vi "EC_Applied_Motion_SXSYSZ_20120115_3ch.vi"() -> ()   [LabVIEW 2015]
uses:
  <vilib>/Utility/file.llb/Read From Spreadsheet File (I64).vi
  <vilib>/Utility/file.llb/Read From Spreadsheet File (string).vi
  <vilib>/Instr/_visa.llb/VISA Configure Serial Port (Instr).vi
  <vilib>/Utility/file.llb/Write To Spreadsheet File (I64).vi
  <vilib>/Utility/file.llb/Write To Spreadsheet File (string).vi
panel:
  out "Z Velocity MV mm/sec":dbl format="%.3f"
  out "Z Position MV mm":dbl
  out "Y Velocity MV mm/sec":dbl format="%.3f"
  out "Y Position MV mm":dbl
  out "X Velocity MV mm/sec":dbl format="%.3f"
  out "X Position MV mm":dbl
  out "Presets":i32[][](array[numeric])
  in  "stop":bool
  in  "Tab Control 3":enum32{"Status", "Reset"}(tab)
  out "Y in Range":bool
  out "Y Scan":bool
  out "Y in Motion":bool
  out "Y Backlash corr":bool
  out "X  in Range":bool
  out "X Scan":bool
  out "X  in Motion":bool
  out "X Backlash corr":bool
  out "Z in Range":bool
  out "Z Scan":bool
  out "Z in Motion":bool
  out "Z Backlash corr":bool
  out "X Ready":bool
  out "Y Ready":bool
  out "Z Ready":bool
  in  "Reset Y Position mm":dbl
  out "Reset Y Motor Steps":i32
  in  "Reset X Position mm":dbl
  out "Reset X Motor Steps":i32
  in  "Reset Z Position mm":dbl
  out "Reset Z Motor Steps":i32
  in  "Reset":bool
  in  "Tab Control 2":enum32{"mm", "step"}(tab)
  in  "X Scan Length SP mm":dbl
  in  "X Scan Velocity SP mm/sec":dbl
  in  "X Scan set":bool
  in  "Y Scan Length SP mm":dbl
  in  "Y Scan Velocity SP mm/sec":dbl
  in  "Y Scan set":bool
  in  "Z Scan Length SP mm":dbl
  in  "Z Scan Velocity SP mm/sec":dbl
  in  "Z Scan set":bool
  in  "X Scan Velocity SP steps/sec":i32=1 min=1 max=102400 step=1
  in  "X Scan Length SP steps":i32 min=-500000 max=500000 step=100
  out "X Scan length MV mm":dbl
  out "X Scan velocity MV mm/sec":dbl format="%#_6f"
  in  "Y Scan Velocity SP steps/sec":i32=1 min=1 max=102400 step=1
  in  "Y Scan Length SP steps":i32 min=-1000000 max=0 step=100
  out "Y Scan length MV mm":dbl
  out "Y Scan velocity MV mm/sec":dbl format="%#_6f"
  in  "Z Scan Velocity SP steps/sec":i32=1 min=1 max=102400 step=1
  in  "Z Scan Length SP steps":i32 min=-204724 max=102195276 step=100
  out "Z Scan length MV mm":dbl
  out "Z Scan velocity MV mm/sec":dbl format="%#_6f"
  out "atan Y/Z":dbl
  in  "Tab Control":enum32{"mm", "preset", "step"}(tab)
  in  "X Position SP mm":dbl
  in  "X Velocity SP mm/sec":dbl
  in  "X Move Set":bool
  in  "Y Move Set":bool
  in  "Y Position SP mm":dbl
  in  "Y Velocity SP mm/sec":dbl
  in  "Z Position SP mm":dbl
  in  "Z Velocity SP mm/sec":dbl
  in  "Z Move Set":bool
  in  "Add Button":bool
  in  "String":string
  in  "Delete Button":bool
  in  "Preset positions":i32(ring) items=["ZERO", "Default", "CDOSE", "QMS", "test", "test2", "test3"]
  in  "Set Button":bool
  in  "X Velocity SP step/sec":i32 min=1 max=50000
  in  "Y Velocity SP step/sec":i32 min=1 max=50000
  in  "Z Velocity SP step/sec":i32 min=1 max=5000
  in  "Y Step SP":i32=-20000 min=-800000 max=800000 step=500
  in  "X Step SP":i32=-20000 min=-750000 max=750000 step=500
  in  "Z Step SP":i32=-20000 min=-3000 max=102400000 step=500
  out "X Step PV":i32 max=2000
  out "Y Step PV":i32 max=2000
  out "Z Step PV":i32 max=2000
  out "R Step PV":i32 max=2000
  out "X Scan Duration":dbl
  out "Y Scan Duration":dbl
  out "Z Scan Duration":dbl
  out "Z COM PORT":refnum<visa-resource-name>="COM5"
  out "Z Backlash steps/sec":i32
  out "Z Backlash":i32
  out "Z Holding Current %":i32
  out "Z Run Current %":i32
  out "Z offset mm":dbl
  out "Z mm/rev":dbl
  out "Z steps/rev":u32
  out "Z  velocity PV step/sec":i32
  out "Z MINPOS":i32=-94296
  out "Z MAXPOS":i32=-34296
  in  "Z Scan OK":bool
  in  "Z Go":bool
  out "Z Position mm PV":dbl
  out "X Position mm PV":dbl
  out "X velocity PV step/sec":i32
  in  "X Scan OK":bool
  in  "X Go":bool
  out "X Backlash steps/sec":i32
  out "X Backlash":i32
  out "X Holding Current %":i32
  out "X Run Current %":i32
  out "X offset mm":dbl
  out "X mm/rev":dbl
  out "X steps/rev":u32
  out "X MAXPOS":i32=-34296
  out "X MINPOS":i32=-94296
  out "X COM PORT":refnum<visa-resource-name>="COM5"
  out "Y Backlash steps/sec":i32
  out "Y Backlash":i32
  out "Y Holding Current %":i32
  out "Y Run Current %":i32
  in  "Scan Cancel":bool
  out "Y Position mm PV":dbl
  out "Y offset mm":dbl
  out "Y mm/rev":dbl
  out "Y steps/rev":u32
  out "Y velocity PV step/sec":i32
  in  "Y Scan OK":bool
  in  "Scan Go":bool
  in  "Stop":bool
  in  "Y Go":bool
  out "Y MINPOS":i32=-94296
  out "Y MAXPOS":i32=-34296
  out "Y COM PORT":refnum<visa-resource-name>="COM5"
  # "REF"
  # "Current position"
  # "Goto position"
  # "RX"
  # "RX"
  # "RY"
  # "RY"
  # "RZ"
  # "RZ"
  # "R,L = green"
  # "L"
  # "M"
  # "B"
  # "S"
  # "R"
  # "Preset position"
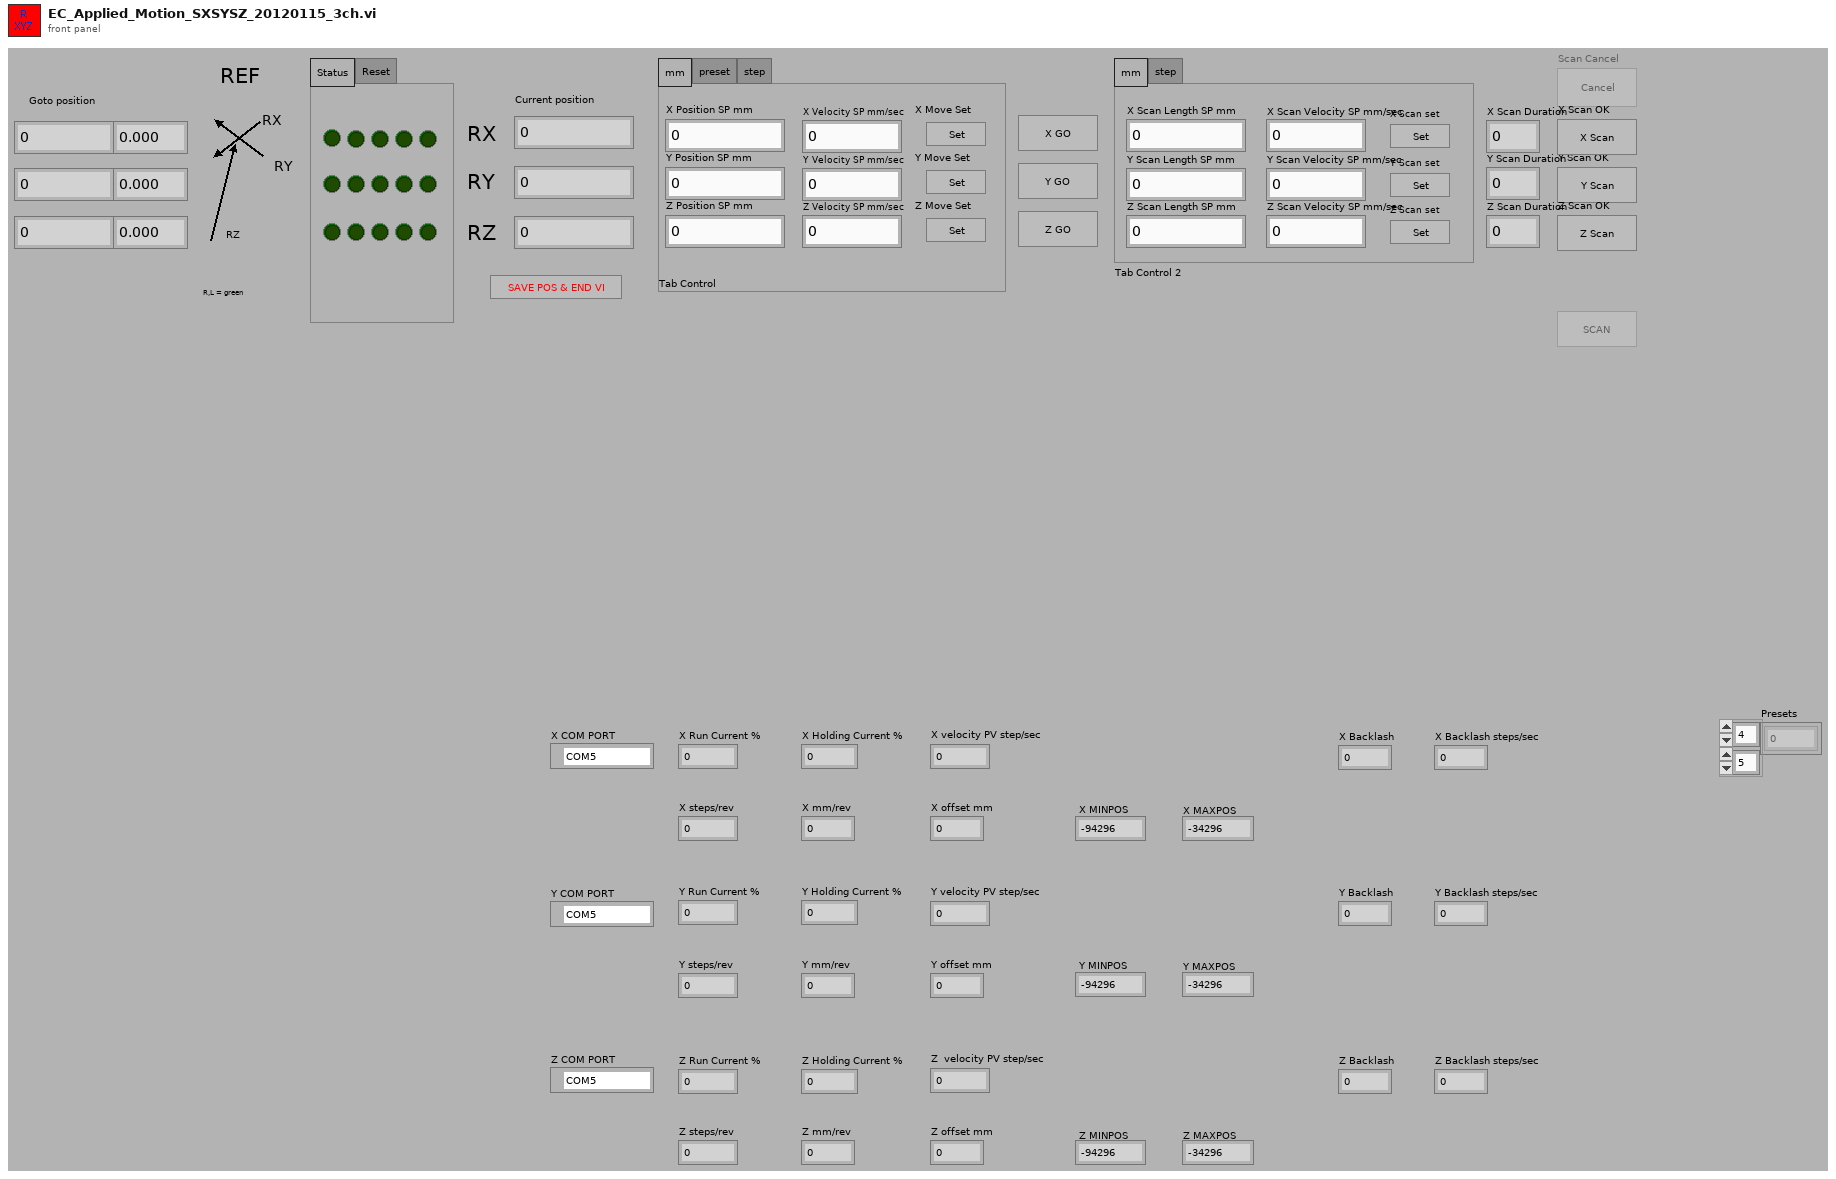
[diagram p1: front panel]
types:
  T1 = enum16{"Power-up Signature", "Accel Rate", "Accel Max", "Bit Rate", "Buffer Status", "Change Current", "Commence Jogging", "Change Jog Speed", "Continue", "Define Address", "Distance for FC,FM,FO,FY", "Decel Rate", "Distance or Position", "Define Limits", "Encoder Deadband", "Encoder Function", "Encoder Position", "Encoder Ratio", "Feed to Length with Speed Change", "Feed to Length", "Feed to Sensor with Mask Dist", "Feed to Length & Set Output", "Feed to Position", "Feed to Sensor", "Feed to Sensor w/safety", "Follow Handwheel", "Immediate Distance?", "Immediate Encoder?", "Immediate Low Output", "Immediate High Output", "Immediate Position?", "Input Status?", "Jog Accel/Decel", "Jog Disable", "Jog Enable", "Jog Speed", "Motor Disable", "Motor Enable", "Microstep Resolution", "Power up Current", "Power up Mode", "Pause", "Request Status", "Revision Level?", "Seek Home", "Stop Jogging", "Stop & Kill Buffer", "Set Output", "Set ABS Position", "Send String", "Stop", "Velocity for Speed Change", "Velocity Setting", "Wait for Input", "Wait Time"}
  T2 = enum8{"Enabled", "Disabled", "Disabled and Grayed Out"}
  T3 = cluster{"first row[0]":i64, "first row[1]":i64, "first row[2]":i64, "first row[3]":i64, "first row[4]":i64, "first row[5]":i64, "first row[6]":i64, "first row[7]":i64, "first row[8]":i64}
  T4 = cluster{"Value[0]":i32, "Value[1]":i32, "Value[2]":i32, "Value[3]":i32, "Value[4]":i32, "Value[5]":i32, "Value[6]":i32, "Value[7]":i32, "Value[8]":i32}
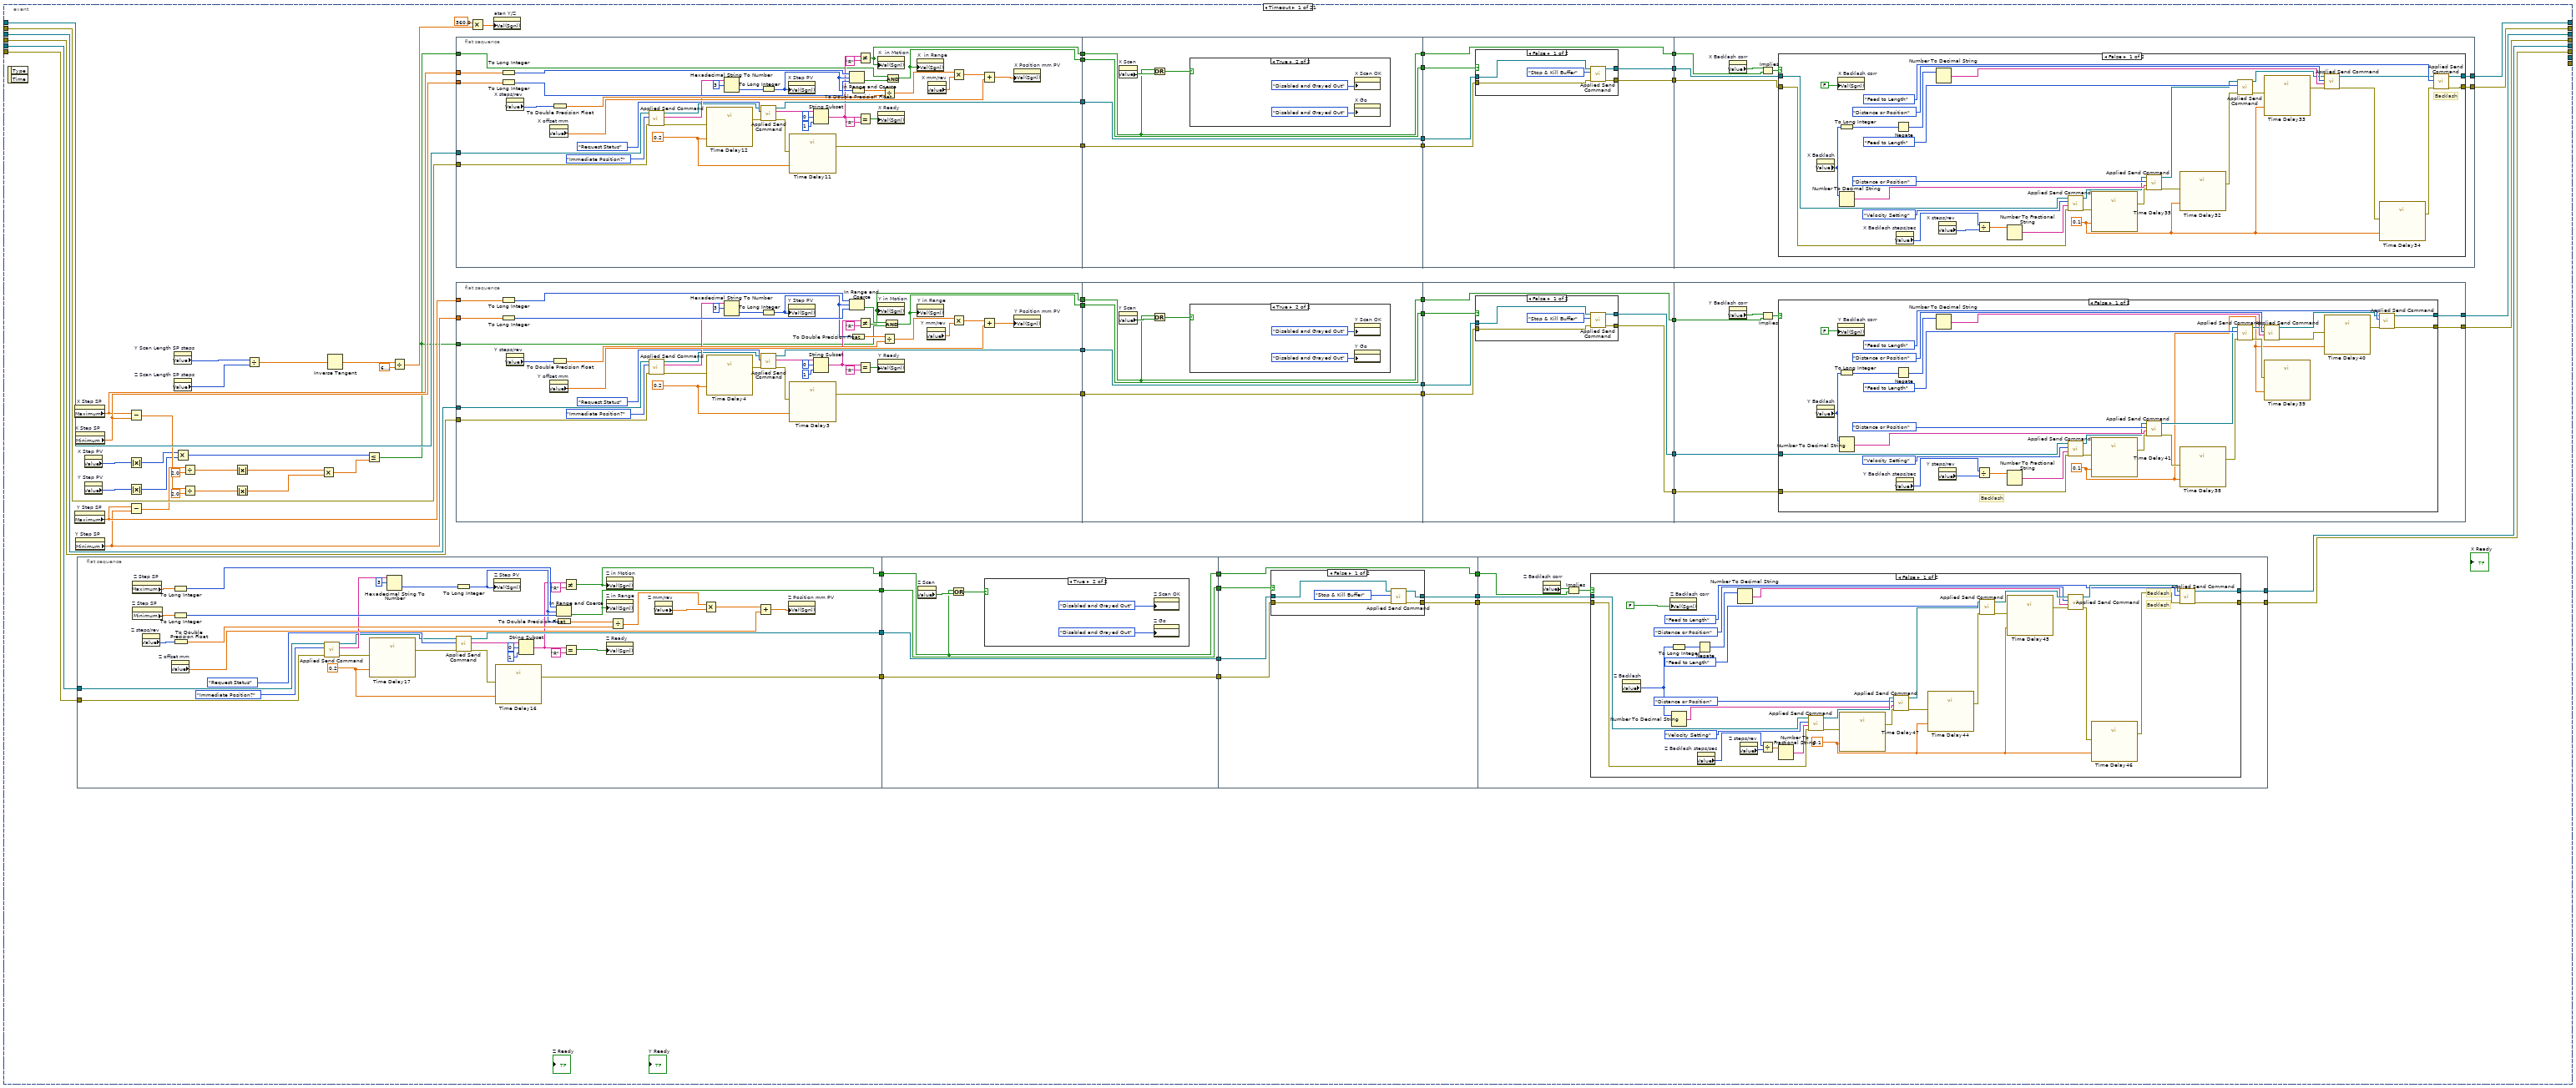
[diagram p5: hidden frame]
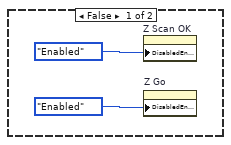
[diagram p6: hidden frame]
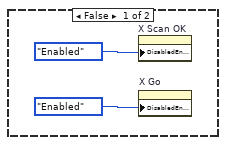
[diagram p9: hidden frame]
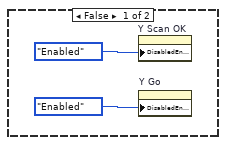
[diagram p12: hidden frame]
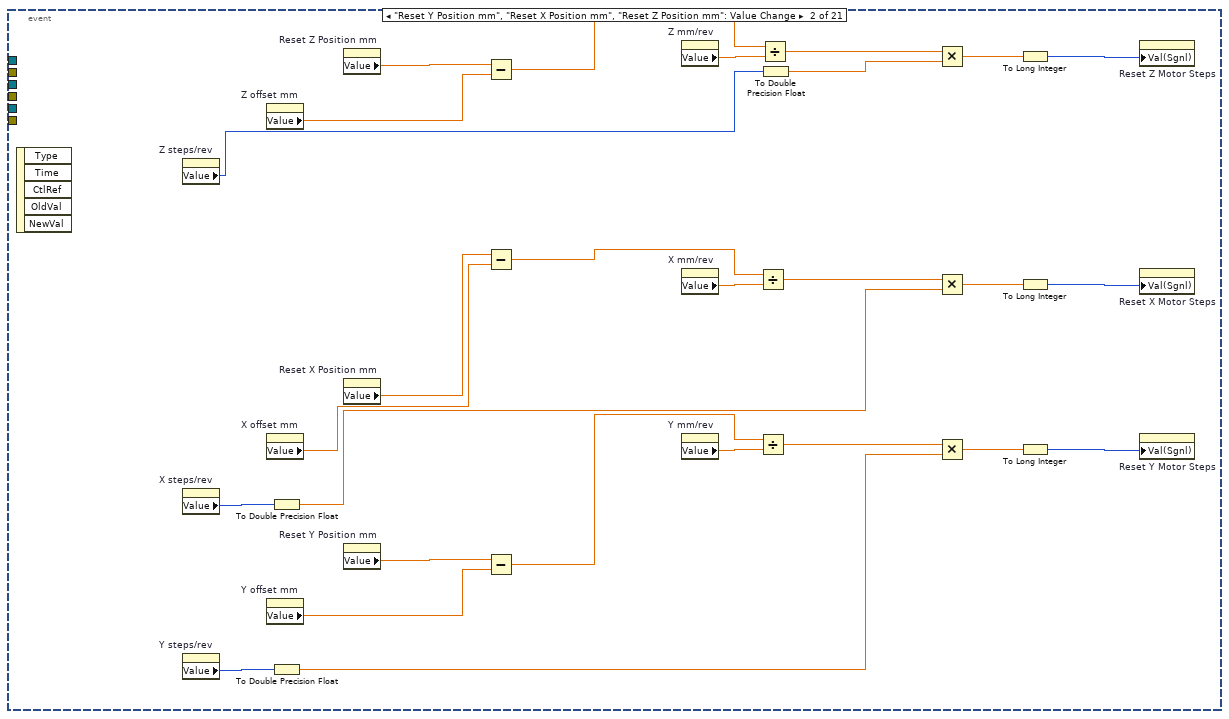
[diagram p15: hidden frame]
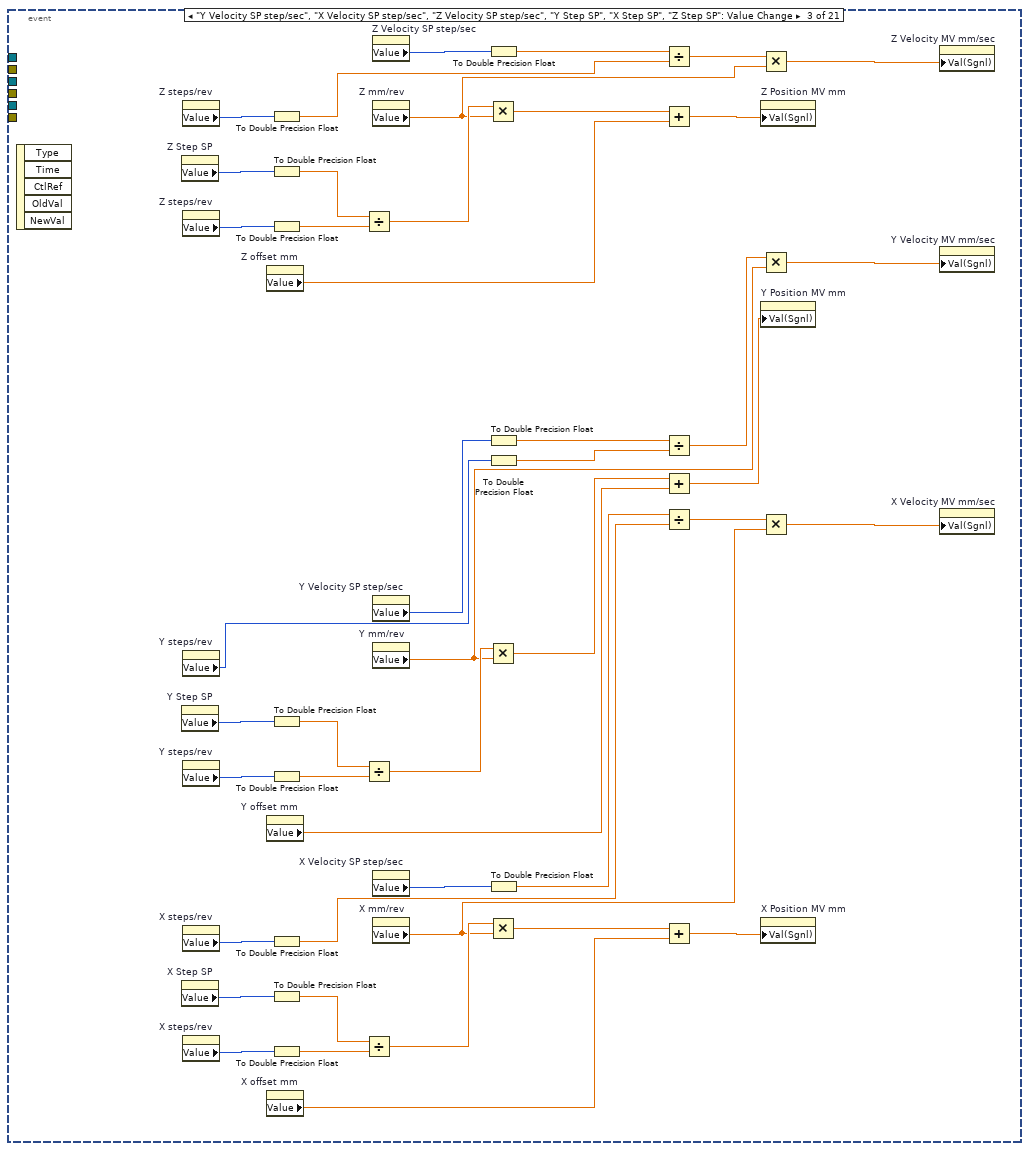
[diagram p16: hidden frame]
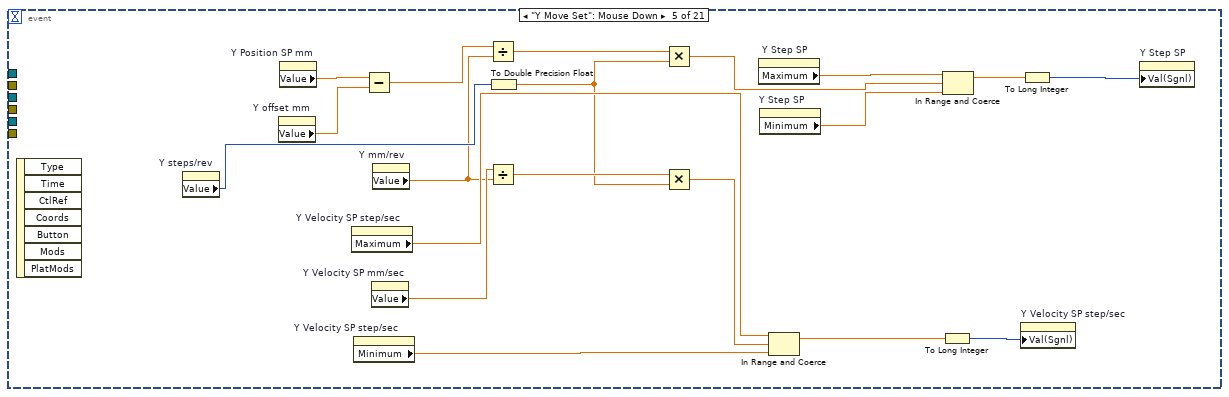
[diagram p17: hidden frame]
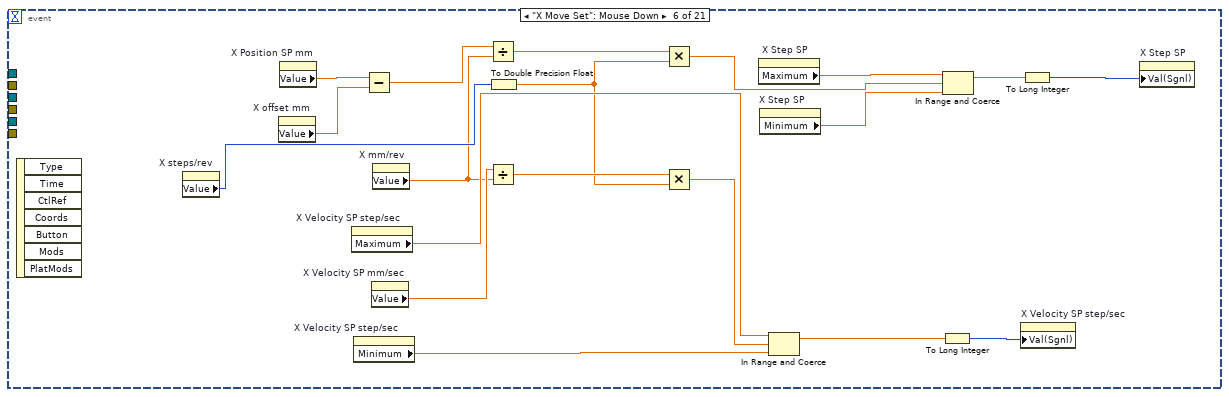
[diagram p18: hidden frame]
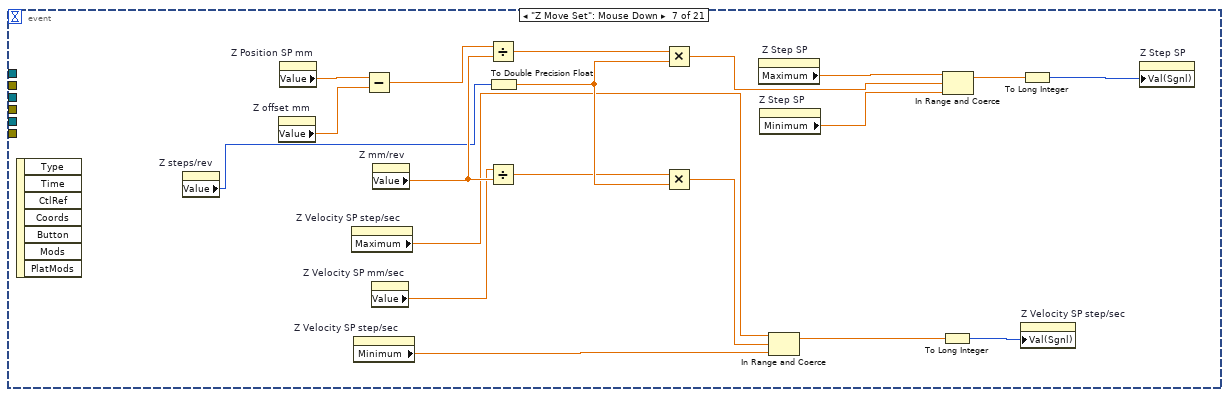
[diagram p19: hidden frame]
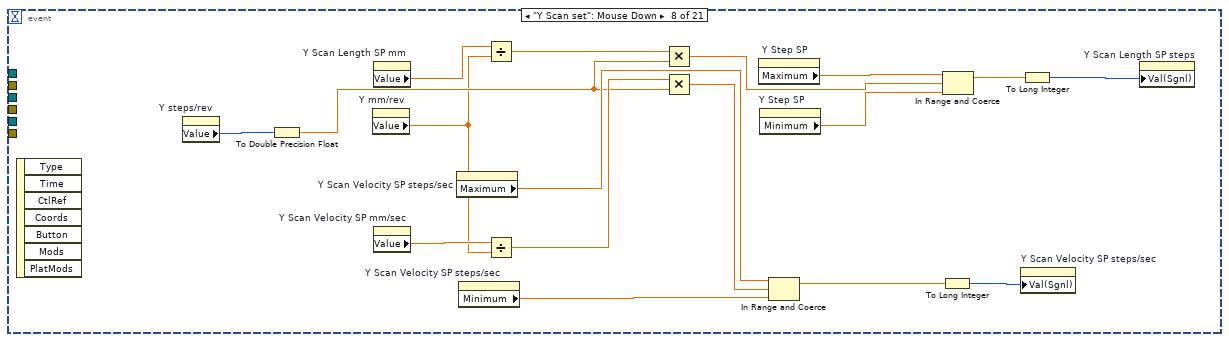
[diagram p20: hidden frame]
diagram:
  (unwired) FALSE
  w19 = 0 ("dimension size")
  n1 = flat-sequence {
    tunnel: [w78] -> w5
    tunnel: [w77] -> w4
    tunnel: w5 -> [w92]
    tunnel: w4 -> [w91]
    tunnel: [w90] -> w3
    tunnel: [w89] -> w2
    tunnel: [w100] -> w49
    tunnel: [w99] -> w48
    tunnel: w3 -> [w102]
    tunnel: w2 -> [w101]
    tunnel: w49 -> [w117]
    tunnel: w48 -> [w116]
    tunnel: [w118] -> w47
    tunnel: [w119] -> w46
    tunnel: [w120] -> w1
    tunnel: [w131] -> w44
    tunnel: [w132] -> w45
    tunnel: w47 -> [w132]
    tunnel: w46 -> [w131]
    tunnel: w1 -> [w129]
    frame #0 {
      "Z Run Current %" <- 100 ("Z Run Current %")
      "Z Holding Current %" <- 50 ("Z Holding Current %")
    }
    frame #1 {
      "Z Backlash steps/sec" <- 1000 ("Z Backlash steps/sec")
      "Z Backlash" <- -2500 ("Z Backlash")
    }
    frame #2 {
      w68 = 2.54 ("Z mm/rev")
      w67 = u32 20000 ("step/rev")
      w69 = 5000 ("Value (Signaling)")
      n2 = property on="Z Velocity SP step/sec" class="DigNum (strict)"("Minimum"=1.0 ("Data Entry Limits:Minimum")) -> ()  [unwired: 2 in, 2 out]
      n3 = property on="Z Scan Velocity SP mm/sec" class="DigNum (strict)"("Val(Sgnl)"=0.1 ("Value (Signaling)")) -> ()  [unwired: 2 in, 2 out]
      n4 = property on="Z Velocity SP step/sec" class="DigNum (strict)"("Val(Sgnl)"=w69) -> ()  [unwired: 2 in, 2 out]
      n5 = To Double Precision Float(number=w69) -> (double precision float=w73:dbl)
      n6 = property on="Z Velocity SP step/sec" class="DigNum (strict)"("Maximum"=w73) -> ()  [unwired: 2 in, 2 out]
      n7 = To Double Precision Float(number=w67) -> (double precision float=w72:dbl)
      n8 = Divide(x=w73, y=w72) -> (x/y=w70:dbl)
      n9 = Multiply(x=w70, y=w68) -> (x*y=w71:dbl)
      n10 = property on="Z Velocity SP mm/sec" class="DigNum (strict)"("Val(Sgnl)"=w71) -> ()  [unwired: 2 in, 2 out]
      "Z mm/rev" <- w68
      "Z steps/rev" <- w67
    }
    frame #3 {
      w75 = -3000 ("lower limit")
      w74 = 102400000 ("upper limit")
      n11 = property on="Z Step SP" class="DigNum (strict)"("Minimum"=w75) -> ()  [unwired: 2 in, 2 out]
      n12 = property on="Z Step SP" class="DigNum (strict)"("Maximum"=w74) -> ()  [unwired: 2 in, 2 out]
      "Z offset mm" <- 0.0 ("Z offset mm")
      "Z MINPOS" <- w75
      "Z MAXPOS" <- w74
    }
    frame #4 {
      w85 = refnum<visa-resource-name> "COM15" ("COM PORT")
      w83 = u16 0 items=["None", "XON/XOFF", "RTS/CTS", "XON/XOFF & RTS/CTS", "DTR/DSR", "XON/XOFF & DTR/DSR"] ("flow control (0:none)")
      w82 = u16 10 items=["1.0"=10, "1.5"=15, "2.0"=20] ("stop bits (10: 1 bit)")
      # "Stop bits"
      n13 = call-poly "VISA Configure Serial Port"("VISA resource name"=w85, "timeout (10sec)"=u32 10000, "baud rate (9600)"=u32 9600, "data bits (8)"=u16 8, "parity (0:none)"=enum16{"None", "Odd", "Even", "Mark", "Space"}."None", "stop bits (10: 1 bit)"=w82, "flow control (0:none)"=w83) -> ("VISA resource name out"=w78:refnum<visa-resource-name>, "error out"=w77:errorcluster)  [unwired: 7 in]
      "Z COM PORT" <- w85
    }
    frame #5 {
      # "Run Current %"
      n14 = property on="Z Run Current %" class="DigNum (strict)"() -> ("Value"=w93:i32)  [unwired: 2 in, 2 out]
      n15 = Divide(x=w93, y=100) -> (x/y=w94:dbl)
      n16 = Multiply(x=w94, y=3.5) -> (x*y=w88:dbl)
      n17 = Number To Fractional String(number=w88) -> (F-format string=w95:string)  [unwired: 3 in]
      n18 = call "Applied Send Command.vi"("error in (no error)"=w91, "Extra"=w95, "Command"=T1."Change Current", "VISA resource name"=w92) -> ("error out"=w89:errorcluster, "VISA resource name out"=w90:refnum<visa-resource-name>)  [unwired: 3 in, 1 out]
    }
    frame #6 {
      # "VELOCITY"
      n19 = property on="Z steps/rev" class="DigNum (strict)"() -> ("Value"=w98:u32)  [unwired: 2 in, 2 out]
      n20 = property on="Z Velocity SP step/sec" class="DigNum (strict)"() -> ("Value"=w97:i32)  [unwired: 2 in, 2 out]
      n21 = Divide(x=w97, y=w98) -> (x/y=w105:dbl)
      n22 = Number To Fractional String(number=w105) -> (F-format string=w107:string)  [unwired: 3 in]
      n23 = call "Applied Send Command.vi"("error in (no error)"=w101, "Extra"=w107, "Command"=T1."Velocity Setting", "VISA resource name"=w102) -> ("error out"=w108:errorcluster, "VISA resource name out"=w115:refnum<visa-resource-name>)  [unwired: 3 in, 1 out]
      n24 = call "Time Delay2"("error in (no error)"=w108, "Delay Time (s)"=0.1) -> ("error out"=w113:errorcluster)  [unwired: 9 in]
      n25 = call "Applied Send Command.vi"("error in (no error)"=w113, "Extra"="", "Command"=T1."Velocity Setting", "VISA resource name"=w115) -> ("error out"=w99:errorcluster, "read buffer"=w111:string, "VISA resource name out"=w100:refnum<visa-resource-name>)  [unwired: 3 in]
      n26 = Fract/Exp String To Number(string=w111, offset=3) -> (number=w106:dbl)  [unwired: 2 in, 1 out]
      n27 = Multiply(x=w106, y=w98) -> (x*y=w103:dbl)
      n28 = property on="Z  velocity PV step/sec" class="DigNum (strict)"("Val(Sgnl)"=w103) -> ()  [unwired: 2 in, 2 out]
    }
    frame #7 {
      # "GET CURRENT POSITION"
      n29 = call "Applied Send Command.vi"("error in (no error)"=w116, "Extra"="", "Command"=T1."Immediate Position?", "VISA resource name"=w117) -> ("error out"=w122:errorcluster, "read buffer"=w124:string, "VISA resource name out"=w118:refnum<visa-resource-name>)  [unwired: 3 in]
      n30 = call "Time Delay8"("error in (no error)"=w122, "Delay Time (s)"=0.1) -> ("error out"=w119:errorcluster)  [unwired: 9 in]
      n31 = Hexadecimal String To Number(string=w124, offset=3) -> (number=w120:u32)  [unwired: 1 in, 1 out]
    }
    frame #8 {
      n32 = property on="Z Step SP" class="DigNum (strict)"() -> ("Maximum"=w128:dbl)  [unwired: 2 in, 2 out]
      n33 = property on="Z Step SP" class="DigNum (strict)"() -> ("Minimum"=w127:dbl)  [unwired: 2 in, 2 out]
      n34 = property on="Z Step SP" class="DigNum (strict)"("Val(Sgnl)"=w129) -> ()  [unwired: 2 in, 2 out]
      n35 = In Range and Coerce(upper limit=w128, x=w129, lower limit=w127) -> (In Range?=w130:bool)  [unwired: 1 out]
      n36 = property on="Z in Range" class="Bool (strict)"("Val(Sgnl)"=w130) -> ()  [unwired: 2 in, 2 out]
    }
  }
  n37 = flat-sequence {
    frame #0 {
      n38 = property on="X Scan" class="Bool (strict)"("Val(Sgnl)"=FALSE ("Value (Signaling)")) -> ()  [unwired: 2 in, 2 out]
      n39 = property on="Y Scan" class="Bool (strict)"("Val(Sgnl)"=FALSE ("Value (Signaling)")) -> ()  [unwired: 2 in, 2 out]
      n40 = property on="Z Scan" class="Bool (strict)"("Val(Sgnl)"=FALSE ("Value (Signaling)")) -> ()  [unwired: 2 in, 2 out]
      n41 = property on="Scan Go" class="Bool"("DisabledEnum"=T2."Disabled and Grayed Out" ("Disabled")) -> ()  [unwired: 2 in, 2 out]
      n42 = property on="Scan Cancel" class="Bool"("DisabledEnum"=T2."Disabled and Grayed Out" ("Disabled")) -> ()  [unwired: 2 in, 2 out]
    }
    frame #1 {
      n43 = property on="Y Backlash corr" class="Bool (strict)"("Val(Sgnl)"=FALSE ("Value (Signaling)")) -> ()  [unwired: 2 in, 2 out]
      n44 = property on="X Backlash corr" class="Bool (strict)"("Val(Sgnl)"=FALSE ("Value (Signaling)")) -> ()  [unwired: 2 in, 2 out]
      n45 = property on="Z Backlash corr" class="Bool (strict)"("Val(Sgnl)"=FALSE ("Value (Signaling)")) -> ()  [unwired: 2 in, 2 out]
    }
  }
  n46 = flat-sequence {
    tunnel: [w158] -> w13
    tunnel: [w157] -> w12
    tunnel: w13 -> [w172]
    tunnel: w12 -> [w171]
    tunnel: [w170] -> w11
    tunnel: [w169] -> w10
    tunnel: w11 -> [w180]
    tunnel: w10 -> [w179]
    tunnel: [w178] -> w9
    tunnel: [w177] -> w8
    tunnel: [w197] -> w53
    tunnel: w9 -> [w200]
    tunnel: w8 -> [w199]
    tunnel: [w198] -> w7
    tunnel: [w196] -> w6
    tunnel: [w209] -> w59
    tunnel: [w212] -> w60
    tunnel: w53 -> [w209]
    tunnel: w7 -> [w212]
    tunnel: w6 -> [w210]
    frame #0 {
      "Y Run Current %" <- 100 ("Run Current %")
      "Y Holding Current %" <- 50 ("Holding Current %")
    }
    frame #1 {
      "Y Backlash" <- 5000 ("Backlash2")
      "Y Backlash steps/sec" <- 10000 ("Value (Signaling)")
    }
    frame #2 {
      w148 = 0.21167 ("MM/rev")
      w151 = u32 20000 ("step/rev")
      w146 = 50000 ("Value (Signaling)")
      n47 = property on="Y Velocity SP step/sec" class="DigNum (strict)"("Minimum"=1.0 ("Data Entry Limits:Minimum")) -> ()  [unwired: 2 in, 2 out]
      n48 = property on="Y Scan Velocity SP mm/sec" class="DigNum (strict)"("Val(Sgnl)"=0.1 ("Value (Signaling)")) -> ()  [unwired: 2 in, 2 out]
      n49 = property on="Y Velocity SP step/sec" class="DigNum (strict)"("Val(Sgnl)"=w146) -> ()  [unwired: 2 in, 2 out]
      n50 = To Double Precision Float(number=w146) -> (double precision float=w152:dbl)
      n51 = property on="Y Velocity SP step/sec" class="DigNum (strict)"("Maximum"=w152) -> ()  [unwired: 2 in, 2 out]
      n52 = To Double Precision Float(number=w151) -> (double precision float=w150:dbl)
      n53 = Divide(x=w152, y=w150) -> (x/y=w147:dbl)
      n54 = Multiply(x=w147, y=w148) -> (x*y=w149:dbl)
      n55 = property on="Y Velocity SP mm/sec" class="DigNum (strict)"("Val(Sgnl)"=w149) -> ()  [unwired: 2 in, 2 out]
      "Y steps/rev" <- w151
      "Y mm/rev" <- w148
    }
    frame #3 {
      w155 = -800000 ("lower limit")
      w156 = 800000 ("upper limit")
      n56 = property on="Y Step SP" class="DigNum (strict)"("Minimum"=w155) -> ()  [unwired: 2 in, 2 out]
      n57 = property on="Y Step SP" class="DigNum (strict)"("Maximum"=w156) -> ()  [unwired: 2 in, 2 out]
      "Y MAXPOS" <- w156
      "Y MINPOS" <- w155
      "Y offset mm" <- 0.0 ("offset")
    }
    frame #4 {
      w165 = refnum<visa-resource-name> "COM14" ("COM PORT")
      w163 = u16 0 items=["None", "XON/XOFF", "RTS/CTS", "XON/XOFF & RTS/CTS", "DTR/DSR", "XON/XOFF & DTR/DSR"] ("flow control (0:none)")
      w162 = u16 10 items=["1.0"=10, "1.5"=15, "2.0"=20] ("stop bits (10: 1 bit)")
      # "Stop bits"
      n58 = call-poly "VISA Configure Serial Port"("VISA resource name"=w165, "timeout (10sec)"=u32 10000, "baud rate (9600)"=u32 9600, "data bits (8)"=u16 8, "parity (0:none)"=enum16{"None", "Odd", "Even", "Mark", "Space"}."None", "stop bits (10: 1 bit)"=w162, "flow control (0:none)"=w163) -> ("VISA resource name out"=w158:refnum<visa-resource-name>, "error out"=w157:errorcluster)  [unwired: 7 in]
      "Y COM PORT" <- w165
    }
    frame #5 {
      n59 = property on="Y Run Current %" class="DigNum (strict)"() -> ("Value"=w173:i32)  [unwired: 2 in, 2 out]
      n60 = Divide(x=w173, y=100) -> (x/y=w174:dbl)
      n61 = Multiply(x=w174, y=3.5) -> (x*y=w168:dbl)
      n62 = Number To Fractional String(number=w168) -> (F-format string=w175:string)  [unwired: 3 in]
      n63 = call "Applied Send Command.vi"("error in (no error)"=w171, "Extra"=w175, "Command"=T1."Change Current", "VISA resource name"=w172) -> ("error out"=w169:errorcluster, "VISA resource name out"=w170:refnum<visa-resource-name>)  [unwired: 3 in, 1 out]
    }
    frame #6 {
      # "VELOCITY"
      n64 = property on="Y steps/rev" class="DigNum (strict)"() -> ("Value"=w184:u32)  [unwired: 2 in, 2 out]
      n65 = property on="Y Velocity SP step/sec" class="DigNum (strict)"() -> ("Value"=w181:i32)  [unwired: 2 in, 2 out]
      n66 = Divide(x=w181, y=w184) -> (x/y=w183:dbl)
      n67 = Number To Fractional String(number=w183) -> (F-format string=w187:string)  [unwired: 3 in]
      n68 = call "Applied Send Command.vi"("error in (no error)"=w179, "Extra"=w187, "Command"=T1."Velocity Setting", "VISA resource name"=w180) -> ("error out"=w188:errorcluster, "VISA resource name out"=w195:refnum<visa-resource-name>)  [unwired: 3 in, 1 out]
      n69 = call "Time Delay36"("error in (no error)"=w188, "Delay Time (s)"=0.1) -> ("error out"=w193:errorcluster)  [unwired: 9 in]
      n70 = call "Applied Send Command.vi"("error in (no error)"=w193, "Extra"="", "Command"=T1."Velocity Setting", "VISA resource name"=w195) -> ("error out"=w177:errorcluster, "read buffer"=w191:string, "VISA resource name out"=w178:refnum<visa-resource-name>)  [unwired: 3 in]
      n71 = Fract/Exp String To Number(string=w191, offset=3) -> (number=w186:dbl)  [unwired: 2 in, 1 out]
      n72 = Multiply(x=w186, y=w184) -> (x*y=w185:dbl)
      n73 = property on="Y velocity PV step/sec" class="DigNum (strict)"("Val(Sgnl)"=w185) -> ()  [unwired: 2 in, 2 out]
    }
    frame #7 {
      # "GET CURRENT POSITION"
      n74 = call "Applied Send Command.vi"("error in (no error)"=w199, "Extra"="", "Command"=T1."Immediate Position?", "VISA resource name"=w200) -> ("error out"=w202:errorcluster, "read buffer"=w204:string, "VISA resource name out"=w198:refnum<visa-resource-name>)  [unwired: 3 in]
      n75 = call "Time Delay37"("error in (no error)"=w202, "Delay Time (s)"=0.1) -> ("error out"=w197:errorcluster)  [unwired: 9 in]
      n76 = Hexadecimal String To Number(string=w204, offset=3) -> (number=w196:u32)  [unwired: 1 in, 1 out]
    }
    frame #8 {
      n77 = property on="Y Step SP" class="DigNum (strict)"() -> ("Maximum"=w208:dbl)  [unwired: 2 in, 2 out]
      n78 = property on="Y Step SP" class="DigNum (strict)"() -> ("Minimum"=w207:dbl)  [unwired: 2 in, 2 out]
      n79 = property on="Y Step SP" class="DigNum (strict)"("Val(Sgnl)"=w210) -> ()  [unwired: 2 in, 2 out]
      n80 = In Range and Coerce(upper limit=w208, x=w210, lower limit=w207) -> (In Range?=w211:bool)  [unwired: 1 out]
      n81 = property on="Y in Range" class="Bool (strict)"("Val(Sgnl)"=w211) -> ()  [unwired: 2 in, 2 out]
    }
  }
  n82 = flat-sequence {
    tunnel: [w230] -> w18
    tunnel: [w229] -> w17
    tunnel: w18 -> [w247]
    tunnel: w17 -> [w246]
    tunnel: [w245] -> w16
    tunnel: [w244] -> w15
    tunnel: [w250] -> w58
    tunnel: w16 -> [w258]
    tunnel: w15 -> [w257]
    tunnel: [w251] -> w14
    tunnel: w58 -> [w272]
    tunnel: [w271] -> w52
    tunnel: [w269] -> w51
    tunnel: [w274] -> w50
    tunnel: w14 -> [w273]
    tunnel: [w283] -> w56
    tunnel: [w284] -> w57
    tunnel: w52 -> [w284]
    tunnel: w51 -> [w283]
    tunnel: w50 -> [w279]
    frame #0 {
      "X Run Current %" <- 100 ("Run Current %")
      "X Holding Current %" <- 50 ("Holding Current %")
    }
    frame #1 {
      "X Backlash steps/sec" <- 10000 ("Value (Signaling)")
      "X Backlash" <- 5000 ("Backlash2")
    }
    frame #2 {
      w219 = 0.21167 ("MM/rev")
      w222 = u32 20000 ("step/rev")
      w217 = 50000 ("Value (Signaling)")
      n83 = property on="X Velocity SP step/sec" class="DigNum (strict)"("Minimum"=1.0 ("Data Entry Limits:Minimum")) -> ()  [unwired: 2 in, 2 out]
      n84 = property on="X Velocity SP step/sec" class="DigNum (strict)"("Val(Sgnl)"=w217) -> ()  [unwired: 2 in, 2 out]
      n85 = property on="X Scan Velocity SP mm/sec" class="DigNum (strict)"("Val(Sgnl)"=0.1 ("Value (Signaling)")) -> ()  [unwired: 2 in, 2 out]
      n86 = To Double Precision Float(number=w217) -> (double precision float=w223:dbl)
      n87 = property on="X Velocity SP step/sec" class="DigNum (strict)"("Maximum"=w223) -> ()  [unwired: 2 in, 2 out]
      n88 = To Double Precision Float(number=w222) -> (double precision float=w221:dbl)
      n89 = Divide(x=w223, y=w221) -> (x/y=w218:dbl)
      n90 = Multiply(x=w218, y=w219) -> (x*y=w220:dbl)
      n91 = property on="X Velocity SP mm/sec" class="DigNum (strict)"("Val(Sgnl)"=w220) -> ()  [unwired: 2 in, 2 out]
      "X steps/rev" <- w222
      "X mm/rev" <- w219
    }
    frame #3 {
      w228 = -750000 ("lower limit")
      w227 = 750000 ("upper limit")
      n92 = property on="X Step SP" class="DigNum (strict)"("Minimum"=w228) -> ()  [unwired: 2 in, 2 out]
      n93 = property on="X Step SP" class="DigNum (strict)"("Maximum"=w227) -> ()  [unwired: 2 in, 2 out]
      "X offset mm" <- 0.0 ("offset")
      "X MAXPOS" <- w227
      "X MINPOS" <- w228
    }
    frame #4 {
      w237 = refnum<visa-resource-name> "COM13" ("COM PORT")
      w235 = u16 0 items=["None", "XON/XOFF", "RTS/CTS", "XON/XOFF & RTS/CTS", "DTR/DSR", "XON/XOFF & DTR/DSR"] ("flow control (0:none)")
      w234 = u16 10 items=["1.0"=10, "1.5"=15, "2.0"=20] ("stop bits (10: 1 bit)")
      # "Stop bits"
      n94 = call-poly "VISA Configure Serial Port"("VISA resource name"=w237, "timeout (10sec)"=u32 10000, "baud rate (9600)"=u32 9600, "data bits (8)"=u16 8, "parity (0:none)"=enum16{"None", "Odd", "Even", "Mark", "Space"}."None", "stop bits (10: 1 bit)"=w234, "flow control (0:none)"=w235) -> ("VISA resource name out"=w230:refnum<visa-resource-name>, "error out"=w229:errorcluster)  [unwired: 7 in]
      "X COM PORT" <- w237
    }
    frame #5 {
      n95 = property on="X Run Current" class="DigNum (strict)"() -> ("Value"=w242:i32)  [unwired: 2 in, 2 out]
      n96 = Divide(x=w242, y=100) -> (x/y=w239:dbl)
      n97 = Multiply(x=3.5 ("y"), y=w239) -> (x*y=w241:dbl)
      n98 = Number To Fractional String(number=w241) -> (F-format string=w243:string)  [unwired: 3 in]
      n99 = call "Applied Send Command.vi"("error in (no error)"=w246, "Extra"=w243, "Command"=T1."Change Current", "VISA resource name"=w247) -> ("error out"=w245:errorcluster, "VISA resource name out"=w244:refnum<visa-resource-name>)  [unwired: 3 in, 1 out]
    }
    frame #6 {
      # "VELOCITY"
      n100 = property on="X steps/rev" class="DigNum (strict)"() -> ("Value"=w253:u32)  [unwired: 2 in, 2 out]
      n101 = property on="X Velocity SP step/sec" class="DigNum (strict)"() -> ("Value"=w254:i32)  [unwired: 2 in, 2 out]
      n102 = Divide(x=w254, y=w253) -> (x/y=w252:dbl)
      n103 = Number To Fractional String(number=w252) -> (F-format string=w259:string)  [unwired: 3 in]
      n104 = call "Applied Send Command.vi"("error in (no error)"=w258, "Extra"=w259, "Command"=T1."Velocity Setting", "VISA resource name"=w257) -> ("error out"=w260:errorcluster, "VISA resource name out"=w267:refnum<visa-resource-name>)  [unwired: 3 in, 1 out]
      n105 = call "Time Delay30"("error in (no error)"=w260, "Delay Time (s)"=0.1) -> ("error out"=w265:errorcluster)  [unwired: 9 in]
      n106 = call "Applied Send Command.vi"("error in (no error)"=w265, "Extra"="", "Command"=T1."Velocity Setting", "VISA resource name"=w267) -> ("error out"=w250:errorcluster, "read buffer"=w263:string, "VISA resource name out"=w251:refnum<visa-resource-name>)  [unwired: 3 in]
      n107 = Fract/Exp String To Number(string=w263, offset=3) -> (number=w256:dbl)  [unwired: 2 in, 1 out]
      n108 = Multiply(x=w256, y=w253) -> (x*y=w255:dbl)
      n109 = property on="X velocity PV step/sec" class="DigNum (strict)"("Val(Sgnl)"=w255) -> ()  [unwired: 2 in, 2 out]
    }
    frame #7 {
      # "GET CURRENT POSITION"
      n110 = call "Applied Send Command.vi"("error in (no error)"=w272, "Extra"="", "Command"=T1."Immediate Position?", "VISA resource name"=w273) -> ("error out"=w270:errorcluster, "read buffer"=w276:string, "VISA resource name out"=w271:refnum<visa-resource-name>)  [unwired: 3 in]
      n111 = call "Time Delay13"("error in (no error)"=w270, "Delay Time (s)"=0.1) -> ("error out"=w269:errorcluster)  [unwired: 9 in]
      n112 = Hexadecimal String To Number(string=w276, offset=3) -> (number=w274:u32)  [unwired: 1 in, 1 out]
    }
    frame #8 {
      n113 = property on="X Step SP" class="DigNum (strict)"() -> ("Maximum"=w282:dbl)  [unwired: 2 in, 2 out]
      n114 = property on="X Step SP" class="DigNum (strict)"() -> ("Minimum"=w281:dbl)  [unwired: 2 in, 2 out]
      n115 = property on="X Step SP" class="DigNum (strict)"("Val(Sgnl)"=w279) -> ()  [unwired: 2 in, 2 out]
      n116 = In Range and Coerce(upper limit=w282, x=w279, lower limit=w281) -> (In Range?=w280:bool)  [unwired: 1 out]
      n117 = property on="X  in Range" class="Bool (strict)"("Val(Sgnl)"=w280) -> ()  [unwired: 2 in, 2 out]
    }
  }
  n118 = call-poly <vilib>:"Read From Spreadsheet File.vi"("file path (dialog if empty)"=path "S:/SSE/SCL2/POS.TXT") -> ("first row"=w36:i64[])  [unwired: 6 in, 4 out]
  n119 = call-poly <vilib>:"Read From Spreadsheet File.vi"("file path (dialog if empty)"=path "S:/SSE/SCL2/PRESET.TXT") -> ("all rows"=w25:string[][])  [unwired: 6 in, 4 out]
  n120 = Array To Cluster(array=w36) -> (cluster=w35:T3)
  n121 = Transpose 2D Array(2D array=w25) -> (transposed array=w26:string[][])
  n122 = Unbundle(w35) -> ("first row[0]"=w33:i64, "first row[1]"=w32:i64, "first row[2]"=w31:i64)  [unwired: 6 out]
  n123 = Delete From Array(array=w26, index (row)=0) -> (deleted portion=w27:string[], array with subset deleted=w29:string[][])  [unwired: 2 in]
  n124 = property on="Reset X Motor Steps" class="DigNum (strict)"("Val(Sgnl)"=w33) -> ()  [unwired: 2 in, 2 out]
  n125 = property on="Reset Y Motor Steps" class="DigNum (strict)"("Val(Sgnl)"=w32) -> ()  [unwired: 2 in, 2 out]
  n126 = property on="Reset Z Motor Steps" class="DigNum (strict)"("Val(Sgnl)"=w31) -> ()  [unwired: 2 in, 2 out]
  n127 = property on="Preset positions" class="Ring (strict)"("Strings []"=w27) -> ()  [unwired: 2 in, 2 out]
  n128 = Transpose 2D Array(2D array=w29) -> (transposed array=w30:string[][])
  n129 = Decimal String To Number(string=w30) -> (number=w28:i32[][])  [unwired: 2 in, 1 out]
  n130 = Initialize Array(w19, w19, 4 ("dimension size")) -> (w22:i32[][])
  n131 = Build Array (concatenate)(w22, w28) -> (→"Presets":i32[][])
  n132 = while {
    tunnel: w60 -> [w301]
    tunnel: w59 -> [w304]
    tunnel: [w305] -> w40
    tunnel: [w303] -> w41
    tunnel: w57 -> [w300]
    tunnel: w56 -> [w299]
    tunnel: [w298] -> w55
    tunnel: [w297] -> w54
    tunnel: w45 -> [w296]
    tunnel: w44 -> [w295]
    tunnel: [w294] -> w43
    tunnel: [w293] -> w42
    tunnel: [w292] -> _
    tunnel: [w291] -> _
    stop <- "stop" stop-if-true
    n133 = flat-sequence {
      frame #0 {
      }
      frame #1 {
      }
    }
    n134 = flat-sequence {
      frame #0 {
      }
      frame #1 {
      }
    }
    n135 = property on="Preset positions" class="Ring (strict)"() -> ("Strings []"=w287:string[])  [unwired: 2 in, 2 out]
    n136 = event shown="[3] \"Y Scan Length SP steps\", \"Y Scan Velocity SP steps/sec\", \"X Scan Velocity SP steps/sec\", \"X Scan Length SP steps\", \"Z Scan Velocity SP steps/sec\", \"Z Scan Length SP steps\": Value Change" {
      selector: _ -> [_ _ _ _ _ _ _ _ _ _ _ _ _ _ _ _ _ _ _ _ _]
      dyn-events: _ -> [_ _ _ _ _ _ _ _ _ _ _ _ _ _ _ _ _ _ _ _ _]
      timeout: 200 -> [_ _ _ _ _ _ _ _ _ _ _ _ _ _ _ _ _ _ _ _ _]
      tunnel: w304 -> [w398 _ _ _ _ _ _ _ _ _ w945 _ _ _ w1175 _ w1242 w1254 w1287 w1353 w1463]
      tunnel: [w397 _ _ _ _ _ _ _ _ _ w951 _ _ _ w1173 _ w1242 w1252 w1289 w1349 w1461] -> w305
      tunnel: w301 -> [w355 _ _ _ _ _ _ _ _ _ w946 _ _ _ w1174 _ w1243 w1255 w1288 w1354 w1464]
      tunnel: [w396 _ _ _ _ _ _ _ _ _ w952 _ _ _ w1170 _ w1243 w1253 w1290 w1350 w1462] -> w303
      tunnel: w300 -> [w354 _ _ _ _ _ _ _ _ _ _ _ w1076 w1136 _ _ _ w1249 w1280 w1356 w1460]
      tunnel: w299 -> [w373 _ _ _ _ _ _ _ _ _ _ _ w1075 w1135 _ _ _ w1248 w1279 w1355 w1459]
      tunnel: [w372 _ _ _ _ _ _ _ _ _ _ _ w1074 w1134 _ _ _ w1251 w1278 w1346 w1458] -> w298
      tunnel: [w371 _ _ _ _ _ _ _ _ _ _ _ w1073 w1133 _ _ _ w1250 w1277 w1345 w1457] -> w297
      tunnel: w296 -> [w356 _ _ _ _ _ _ _ _ _ _ w1008 _ _ _ w1208 _ w1247 w1274 w1352 w1456]
      tunnel: w295 -> [w359 _ _ _ _ _ _ _ _ _ _ w1007 _ _ _ w1207 _ w1246 w1273 w1351 w1455]
      tunnel: [w358 _ _ _ _ _ _ _ _ _ _ w1005 _ _ _ w1205 _ w1245 w1272 w1348 _] -> w294
      tunnel: [w357 _ _ _ _ _ _ _ _ _ _ w1006 _ _ _ w1206 _ w1244 w1271 w1347 _] -> w293
      tunnel: [_ _ _ _ _ _ _ _ _ _ _ _ _ _ _ _ _ _ _ _ w1454] -> w292
      tunnel: [_ _ _ _ _ _ _ _ _ _ _ _ _ _ _ _ _ _ _ _ w1453] -> w291
      event Timeout {
        n137 = event-data() -> ()  [unwired: 1 in, 2 out]
        n138 = property on="X Step SP" class="DigNum (strict)"() -> ("Maximum"=w338:dbl)  [unwired: 2 in, 2 out]
        n139 = property on="Y Step SP" class="DigNum (strict)"() -> ("Maximum"=w343:dbl)  [unwired: 2 in, 2 out]
        n140 = property on="X Step SP" class="DigNum (strict)"() -> ("Minimum"=w339:dbl)  [unwired: 2 in, 2 out]
        n141 = property on="Y Step SP" class="DigNum (strict)"() -> ("Minimum"=w342:dbl)  [unwired: 2 in, 2 out]
        n142 = flat-sequence {
          tunnel: [w407] -> w370
          tunnel: [w420] -> w369
          tunnel: [w430] -> w368
          tunnel: [w400] -> w367
          tunnel: w356 -> [w415]
          tunnel: w359 -> [w416]
          tunnel: w370 -> [w440]
          tunnel: [w440] -> w366
          tunnel: w369 -> [w439]
          tunnel: [w439] -> w365
          tunnel: w368 -> [w438]
          tunnel: [w438] -> w364
          tunnel: w367 -> [w435]
          tunnel: [w435] -> w363
          tunnel: w366 -> [w447]
          tunnel: [w448] -> w362
          tunnel: w365 -> [w450]
          tunnel: [w449] -> w361
          tunnel: w364 -> [w446]
          tunnel: [w445] -> w360
          tunnel: w363 -> [w445]
          tunnel: w362 -> [w460]
          tunnel: w361 -> [w461]
          tunnel: w360 -> [w463]
          tunnel: [w459] -> w357
          tunnel: [w458] -> w358
          frame #0 {
            w419 = 0.2 ("Delay Time (s)")
            n143 = property on="Z Step SP" class="DigNum (strict)"() -> ("Maximum"=w432:dbl)  [unwired: 2 in, 2 out]
            n144 = property on="Z Step SP" class="DigNum (strict)"() -> ("Minimum"=w434:dbl)  [unwired: 2 in, 2 out]
            n145 = property on="Z steps/rev" class="DigNum (strict)"() -> ("Value"=w428:u32)  [unwired: 2 in, 2 out]
            n146 = property on="Z offset mm" class="DigNum (strict)"() -> ("Value"=w424:dbl)  [unwired: 2 in, 2 out]
            n147 = To Long Integer(number=w432) -> (32bit integer=w431:i32)
            n148 = To Long Integer(number=w434) -> (32bit integer=w433:i32)
            n149 = To Double Precision Float(number=w428) -> (double precision float=w429:dbl)
            n150 = call "Applied Send Command.vi"("error in (no error)"=w416, "Command"=T1."Immediate Position?", "VISA resource name"=w415) -> ("error out"=w414:errorcluster, "read buffer"=w411:string, "VISA resource name out"=w409:refnum<visa-resource-name>)  [unwired: 4 in]
            n151 = call "Time Delay17"("error in (no error)"=w414, "Delay Time (s)"=w419) -> ("error out"=w399:errorcluster)  [unwired: 9 in]
            n152 = Hexadecimal String To Number(string=w411, offset=3) -> (number=w412:u32)  [unwired: 1 in, 1 out]
            n153 = To Long Integer(number=w412) -> (32bit integer=w422:i32)
            n154 = call "Applied Send Command.vi"("error in (no error)"=w399, "Command"=T1."Request Status", "VISA resource name"=w409) -> ("error out"=w408:errorcluster, "read buffer"=w404:string, "VISA resource name out"=w407:refnum<visa-resource-name>)  [unwired: 4 in]
            n155 = property on="Z Step PV" class="DigNum (strict)"("Val(Sgnl)"=w422) -> ()  [unwired: 2 in, 2 out]
            n156 = call "Time Delay16"("error in (no error)"=w408, "Delay Time (s)"=w419) -> ("error out"=w420:errorcluster)  [unwired: 9 in]
            n157 = String Subset(string=w404, offset (0)=0, length (rest)=1 ("length (rest)")) -> (substring=w401:string)
            n158 = In Range and Coerce(upper limit=w431, x=w422, lower limit=w433) -> (In Range?=w430:bool)  [unwired: 1 out]
            n159 = To Double Precision Float(number=w422) -> (double precision float=w423:dbl)
            n160 = Not Equal?(x=w401, y="R") -> (x != y?=w400:bool)
            n161 = Equal?(x=w401, y="R") -> (x = y?=w418:bool)
            n162 = property on="Z in Motion" class="Bool (strict)"("Val(Sgnl)"=w400) -> ()  [unwired: 2 in, 2 out]
            n163 = property on="Z in Range" class="Bool (strict)"("Val(Sgnl)"=w430) -> ()  [unwired: 2 in, 2 out]
            n164 = property on="Z Ready" class="Bool (strict)"("Val(Sgnl)"=w418) -> ()  [unwired: 2 in, 2 out]
            n165 = Divide(x=w423, y=w429) -> (x/y=w427:dbl)
            n166 = property on="Z mm/rev" class="DigNum (strict)"() -> ("Value"=w426:dbl)  [unwired: 2 in, 2 out]
            n167 = Multiply(x=w427, y=w426) -> (x*y=w425:dbl)
            n168 = Add(x=w425, y=w424) -> (x+y=w421:dbl)
            n169 = property on="Z Position mm PV" class="DigNum (strict)"("Val(Sgnl)"=w421) -> ()  [unwired: 2 in, 2 out]
          }
          frame #1 {
            n170 = property on="Z Scan" class="Bool (strict)"() -> ("Value"=w436:bool)  [unwired: 2 in, 2 out]
            n171 = Or(x=w435, y=w436) -> (x .or. y?=w437:bool)
            n172 = case shown="True" w437 {
              frame False {
                n173 = property on="Z Scan OK" class="Bool"("DisabledEnum"=T2."Enabled" ("Disabled")) -> ()  [unwired: 2 in, 2 out]
                n174 = property on="Z Go" class="Bool"("DisabledEnum"=T2."Enabled" ("Disabled")) -> ()  [unwired: 2 in, 2 out]
              }
              frame True {
                n175 = property on="Z Scan OK" class="Bool"("DisabledEnum"=T2."Disabled and Grayed Out" ("Disabled")) -> ()  [unwired: 2 in, 2 out]
                n176 = property on="Z Go" class="Bool"("DisabledEnum"=T2."Disabled and Grayed Out" ("Disabled")) -> ()  [unwired: 2 in, 2 out]
              }
            }
          }
          frame #2 {
            n177 = case shown="False" w446 {
              tunnel: w447 -> [w454 w457]
              tunnel: [w452 w457] -> w448
              tunnel: [w451 w456] -> w449
              tunnel: w450 -> [w453 w456]
              frame False {
                n178 = call "Applied Send Command.vi"("error in (no error)"=w453, "Command"=T1."Stop & Kill Buffer", "VISA resource name"=w454) -> ("error out"=w451:errorcluster, "VISA resource name out"=w452:refnum<visa-resource-name>)  [unwired: 4 in, 1 out]
              }
              frame True {
              }
            }
          }
          frame #3 {
            n179 = property on="Z Backlash corr" class="Bool (strict)"() -> ("Value"=w464:bool)  [unwired: 2 in, 2 out]
            n180 = Implies(1:w463, 2:w464) -> (0:w462:bool)
            n181 = case shown="False" w462 {
              tunnel: w461 -> [w465 w497]
              tunnel: w460 -> [w466 w498]
              tunnel: [w467 w497] -> w459
              tunnel: [w468 w498] -> w458
              frame False {
                w494 = 0.1 ("Delay Time (s)")
                # "Backlash"
                # "Backlash"
                n182 = property on="Z Backlash" class="DigNum (strict)"() -> ("Value"=w472:i32)  [unwired: 2 in, 2 out]
                n183 = property on="Z Backlash corr" class="Bool (strict)"("Val(Sgnl)"=FALSE ("Value (Signaling)")) -> ()  [unwired: 2 in, 2 out]
                n184 = To Long Integer(number=w472) -> (32bit integer=w475:i32)
                n185 = Number To Decimal String(number=w472) -> (decimal integer string=w480:string)  [unwired: 1 in]
                n186 = Negate(x=w475) -> (-x=w474:i32)
                n187 = property on="Z Backlash steps/sec" class="DigNum (strict)"() -> ("Value"=w471:i32)  [unwired: 2 in, 2 out]
                n188 = Number To Decimal String(number=w474) -> (decimal integer string=w481:string)  [unwired: 1 in]
                n189 = property on="Z steps/rev" class="DigNum (strict)"() -> ("Value"=w470:u32)  [unwired: 2 in, 2 out]
                n190 = Divide(x=w471, y=w470) -> (x/y=w495:dbl)
                n191 = Number To Fractional String(number=w495) -> (F-format string=w496:string)  [unwired: 3 in]
                n192 = call "Applied Send Command.vi"("error in (no error)"=w465, "Extra"=w496, "Command"=T1."Velocity Setting", "VISA resource name"=w466) -> ("error out"=w492:errorcluster, "VISA resource name out"=w485:refnum<visa-resource-name>)  [unwired: 3 in, 1 out]
                n193 = call "Time Delay47"("error in (no error)"=w492, "Delay Time (s)"=w494) -> ("error out"=w493:errorcluster)  [unwired: 9 in]
                n194 = call "Applied Send Command.vi"("error in (no error)"=w493, "Extra"=w480, "Command"=T1."Distance or Position", "VISA resource name"=w485) -> ("error out"=w486:errorcluster, "VISA resource name out"=w479:refnum<visa-resource-name>)  [unwired: 3 in, 1 out]
                n195 = call "Time Delay44"("error in (no error)"=w486, "Delay Time (s)"=w494) -> ("error out"=w487:errorcluster)  [unwired: 9 in]
                n196 = call "Applied Send Command.vi"("error in (no error)"=w487, "Command"=T1."Feed to Length", "VISA resource name"=w479) -> ("error out"=w488:errorcluster, "VISA resource name out"=w482:refnum<visa-resource-name>)  [unwired: 4 in, 1 out]
                n197 = call "Time Delay45"("error in (no error)"=w488, "Delay Time (s)"=w494) -> ("error out"=w489:errorcluster)  [unwired: 9 in]
                n198 = call "Applied Send Command.vi"("error in (no error)"=w489, "Extra"=w481, "Command"=T1."Distance or Position", "VISA resource name"=w482) -> ("error out"=w490:errorcluster, "VISA resource name out"=w483:refnum<visa-resource-name>)  [unwired: 3 in, 1 out]
                n199 = call "Time Delay46"("error in (no error)"=w490, "Delay Time (s)"=w494) -> ("error out"=w491:errorcluster)  [unwired: 9 in]
                n200 = call "Applied Send Command.vi"("error in (no error)"=w491, "Command"=T1."Feed to Length", "VISA resource name"=w483) -> ("error out"=w467:errorcluster, "VISA resource name out"=w468:refnum<visa-resource-name>)  [unwired: 4 in, 1 out]
              }
              frame True {
              }
            }
          }
        }
        n201 = property on="X Step PV" class="DigNum (strict)"() -> ("Value"=w337:i32)  [unwired: 2 in, 2 out]
        n202 = property on="Y Step PV" class="DigNum (strict)"() -> ("Value"=w336:i32)  [unwired: 2 in, 2 out]
        n203 = Subtract(x=w338, y=w339) -> (x-y=w340:dbl)
        n204 = Absolute Value(x=w337) -> (abs(x)=w334:i32)
        n205 = Absolute Value(x=w336) -> (abs(x)=w335:i32)
        n206 = Subtract(x=w343, y=w342) -> (x-y=w344:dbl)
        n207 = property on="Y Scan Length SP steps" class="DigNum (strict)"() -> ("Value"=w346:i32)  [unwired: 2 in, 2 out]
        n208 = property on="Z Scan Length SP steps" class="DigNum (strict)"() -> ("Value"=w347:i32)  [unwired: 2 in, 2 out]
        n209 = Multiply(x=w334, y=w335) -> (x*y=w329:i32)
        n210 = Divide(x=w344, y=2.0) -> (x/y=w332:dbl)
        n211 = Divide(x=w340, y=2.0) -> (x/y=w333:dbl)
        n212 = Absolute Value(x=w332) -> (abs(x)=w330:dbl)
        n213 = Absolute Value(x=w333) -> (abs(x)=w331:dbl)
        n214 = Divide(x=w346, y=w347) -> (x/y=w348:dbl)
        n215 = Multiply(x=w330, y=w331) -> (x*y=w328:dbl)
        n216 = Inverse Tangent(1:w348) -> (0:w349:dbl)
        n217 = Less Or Equal?(x=w329, y=w328) -> (x <= y?=w327:bool)
        n218 = Divide(x=w349, y=6.283185307179586) -> (x/y=w350:dbl)
        n219 = flat-sequence {
          tunnel: [w511] -> w384
          tunnel: [w522] -> w383
          tunnel: [w500] -> w382
          tunnel: [w507] -> w381
          tunnel: w354 -> [w518]
          tunnel: w373 -> [w506]
          tunnel: w338 -> [w502]
          tunnel: w339 -> [w501]
          tunnel: w327 -> [w499]
          tunnel: w384 -> [w542]
          tunnel: [w542] -> w380
          tunnel: w383 -> [w541]
          tunnel: [w541] -> w379
          tunnel: w382 -> [w540]
          tunnel: [w540] -> w378
          tunnel: w381 -> [w537]
          tunnel: [w537] -> w377
          tunnel: w380 -> [w551]
          tunnel: [w548] -> w376
          tunnel: w379 -> [w550]
          tunnel: [w549] -> w375
          tunnel: w378 -> [w547]
          tunnel: [w552] -> w374
          tunnel: w377 -> [w552]
          tunnel: w376 -> [w563]
          tunnel: w375 -> [w564]
          tunnel: w374 -> [w565]
          tunnel: [w562] -> w371
          tunnel: [w561] -> w372
          frame #0 {
            w521 = 0.2 ("Delay Time (s)")
            n220 = To Long Integer(number=w502) -> (32bit integer=w534:i32)
            n221 = To Long Integer(number=w501) -> (32bit integer=w535:i32)
            n222 = property on="X steps/rev" class="DigNum (strict)"() -> ("Value"=w531:u32)  [unwired: 2 in, 2 out]
            n223 = property on="X offset mm" class="DigNum (strict)"() -> ("Value"=w527:dbl)  [unwired: 2 in, 2 out]
            n224 = To Double Precision Float(number=w531) -> (double precision float=w532:dbl)
            n225 = call "Applied Send Command.vi"("error in (no error)"=w506, "Command"=T1."Immediate Position?", "VISA resource name"=w518) -> ("error out"=w516:errorcluster, "read buffer"=w517:string, "VISA resource name out"=w512:refnum<visa-resource-name>)  [unwired: 4 in]
            n226 = call "Time Delay12"("error in (no error)"=w516, "Delay Time (s)"=w521) -> ("error out"=w509:errorcluster)  [unwired: 9 in]
            n227 = Hexadecimal String To Number(string=w517, offset=3) -> (number=w523:u32)  [unwired: 1 in, 1 out]
            n228 = To Long Integer(number=w523) -> (32bit integer=w525:i32)
            n229 = call "Applied Send Command.vi"("error in (no error)"=w509, "Command"=T1."Request Status", "VISA resource name"=w512) -> ("error out"=w510:errorcluster, "read buffer"=w514:string, "VISA resource name out"=w511:refnum<visa-resource-name>)  [unwired: 4 in]
            n230 = property on="X Step PV" class="DigNum (strict)"("Val(Sgnl)"=w525) -> ()  [unwired: 2 in, 2 out]
            n231 = call "Time Delay11"("error in (no error)"=w510, "Delay Time (s)"=w521) -> ("error out"=w522:errorcluster)  [unwired: 9 in]
            n232 = String Subset(string=w514, offset (0)=0, length (rest)=1 ("length (rest)")) -> (substring=w503:string)
            n233 = In Range and Coerce(upper limit=w534, x=w525, lower limit=w535) -> (In Range?=w533:bool)  [unwired: 1 out]
            n234 = To Double Precision Float(number=w525) -> (double precision float=w526:dbl)
            n235 = Not Equal?(x=w503, y="R") -> (x != y?=w507:bool)
            n236 = Equal?(x=w503, y="R") -> (x = y?=w520:bool)
            n237 = property on="X  in Motion" class="Bool (strict)"("Val(Sgnl)"=w507) -> ()  [unwired: 2 in, 2 out]
            n238 = property on="X Ready" class="Bool (strict)"("Val(Sgnl)"=w520) -> ()  [unwired: 2 in, 2 out]
            n239 = Divide(x=w526, y=w532) -> (x/y=w530:dbl)
            n240 = And(x=w499, y=w533) -> (x .and. y?=w500:bool)
            n241 = property on="X  in Range" class="Bool (strict)"("Val(Sgnl)"=w500) -> ()  [unwired: 2 in, 2 out]
            n242 = property on="X mm/rev" class="DigNum (strict)"() -> ("Value"=w529:dbl)  [unwired: 2 in, 2 out]
            n243 = Multiply(x=w530, y=w529) -> (x*y=w528:dbl)
            n244 = Add(x=w528, y=w527) -> (x+y=w524:dbl)
            n245 = property on="X Position mm PV" class="DigNum (strict)"("Val(Sgnl)"=w524) -> ()  [unwired: 2 in, 2 out]
          }
          frame #1 {
            n246 = property on="X Scan" class="Bool (strict)"() -> ("Value"=w538:bool)  [unwired: 2 in, 2 out]
            n247 = Or(x=w537, y=w538) -> (x .or. y?=w539:bool)
            n248 = case shown="True" w539 {
              frame False {
                n249 = property on="X Scan OK" class="Bool"("DisabledEnum"=T2."Enabled" ("Disabled")) -> ()  [unwired: 2 in, 2 out]
                n250 = property on="X Go" class="Bool"("DisabledEnum"=T2."Enabled" ("Disabled")) -> ()  [unwired: 2 in, 2 out]
              }
              frame True {
                n251 = property on="X Scan OK" class="Bool"("DisabledEnum"=T2."Disabled and Grayed Out" ("Disabled")) -> ()  [unwired: 2 in, 2 out]
                n252 = property on="X Go" class="Bool"("DisabledEnum"=T2."Disabled and Grayed Out" ("Disabled")) -> ()  [unwired: 2 in, 2 out]
              }
            }
          }
          frame #2 {
            n253 = case shown="False" w547 {
              tunnel: w551 -> [w554 w559]
              tunnel: [w556 w559] -> w548
              tunnel: [w557 w558] -> w549
              tunnel: w550 -> [w553 w558]
              frame False {
                n254 = call "Applied Send Command.vi"("error in (no error)"=w553, "Command"=T1."Stop & Kill Buffer", "VISA resource name"=w554) -> ("error out"=w557:errorcluster, "VISA resource name out"=w556:refnum<visa-resource-name>)  [unwired: 4 in, 1 out]
              }
              frame True {
              }
            }
          }
          frame #3 {
            n255 = property on="X Backlash corr" class="Bool (strict)"() -> ("Value"=w566:bool)  [unwired: 2 in, 2 out]
            n256 = Implies(1:w565, 2:w566) -> (0:w560:bool)
            n257 = case shown="False" w560 {
              tunnel: w564 -> [w580 w599]
              tunnel: w563 -> [w581 w600]
              tunnel: [w583 w599] -> w562
              tunnel: [w582 w600] -> w561
              frame False {
                w571 = 0.1 ("Delay Time (s)")
                # "Backlash"
                n258 = property on="X Backlash" class="DigNum (strict)"() -> ("Value"=w586:i32)  [unwired: 2 in, 2 out]
                n259 = property on="X Backlash corr" class="Bool (strict)"("Val(Sgnl)"=FALSE ("Value (Signaling)")) -> ()  [unwired: 2 in, 2 out]
                n260 = To Long Integer(number=w586) -> (32bit integer=w595:i32)
                n261 = Number To Decimal String(number=w586) -> (decimal integer string=w590:string)  [unwired: 1 in]
                n262 = Negate(x=w595) -> (-x=w596:i32)
                n263 = property on="X Backlash steps/sec" class="DigNum (strict)"() -> ("Value"=w570:i32)  [unwired: 2 in, 2 out]
                n264 = Number To Decimal String(number=w596) -> (decimal integer string=w589:string)  [unwired: 1 in]
                n265 = property on="X steps/rev" class="DigNum (strict)"() -> ("Value"=w569:u32)  [unwired: 2 in, 2 out]
                n266 = Divide(x=w570, y=w569) -> (x/y=w568:dbl)
                n267 = Number To Fractional String(number=w568) -> (F-format string=w567:string)  [unwired: 3 in]
                n268 = call "Applied Send Command.vi"("error in (no error)"=w580, "Extra"=w567, "Command"=T1."Velocity Setting", "VISA resource name"=w581) -> ("error out"=w573:errorcluster, "VISA resource name out"=w584:refnum<visa-resource-name>)  [unwired: 3 in, 1 out]
                n269 = call "Time Delay35"("error in (no error)"=w573, "Delay Time (s)"=w571) -> ("error out"=w572:errorcluster)  [unwired: 9 in]
                n270 = call "Applied Send Command.vi"("error in (no error)"=w572, "Extra"=w590, "Command"=T1."Distance or Position", "VISA resource name"=w584) -> ("error out"=w579:errorcluster, "VISA resource name out"=w591:refnum<visa-resource-name>)  [unwired: 3 in, 1 out]
                n271 = call "Time Delay32"("error in (no error)"=w579, "Delay Time (s)"=w571) -> ("error out"=w578:errorcluster)  [unwired: 9 in]
                n272 = call "Applied Send Command.vi"("error in (no error)"=w578, "Command"=T1."Feed to Length", "VISA resource name"=w591) -> ("error out"=w577:errorcluster, "VISA resource name out"=w588:refnum<visa-resource-name>)  [unwired: 4 in, 1 out]
                n273 = call "Time Delay33"("error in (no error)"=w577, "Delay Time (s)"=w571) -> ("error out"=w576:errorcluster)  [unwired: 9 in]
                n274 = call "Applied Send Command.vi"("error in (no error)"=w576, "Extra"=w589, "Command"=T1."Distance or Position", "VISA resource name"=w588) -> ("error out"=w575:errorcluster, "VISA resource name out"=w587:refnum<visa-resource-name>)  [unwired: 3 in, 1 out]
                n275 = call "Time Delay34"("error in (no error)"=w575, "Delay Time (s)"=w571) -> ("error out"=w574:errorcluster)  [unwired: 9 in]
                n276 = call "Applied Send Command.vi"("error in (no error)"=w574, "Command"=T1."Feed to Length", "VISA resource name"=w587) -> ("error out"=w583:errorcluster, "VISA resource name out"=w582:refnum<visa-resource-name>)  [unwired: 4 in, 1 out]
              }
              frame True {
              }
            }
          }
        }
        n277 = flat-sequence {
          tunnel: w398 -> [w617]
          tunnel: w355 -> [w618]
          tunnel: [w614] -> w395
          tunnel: [w624] -> w393
          tunnel: [w603] -> w391
          tunnel: [w605] -> w389
          tunnel: w343 -> [w604]
          tunnel: w342 -> [w601]
          tunnel: w327 -> [w602]
          tunnel: w395 -> [w644]
          tunnel: [w644] -> w394
          tunnel: w393 -> [w643]
          tunnel: [w643] -> w392
          tunnel: w391 -> [w642]
          tunnel: [w642] -> w390
          tunnel: w389 -> [w639]
          tunnel: [w639] -> w385
          tunnel: w394 -> [w651]
          tunnel: [w652] -> w388
          tunnel: w392 -> [w654]
          tunnel: [w653] -> w387
          tunnel: w390 -> [w650]
          tunnel: [w649] -> w386
          tunnel: w385 -> [w649]
          tunnel: w388 -> [w664]
          tunnel: w387 -> [w665]
          tunnel: w386 -> [w667]
          tunnel: [w663] -> w397
          tunnel: [w662] -> w396
          frame #0 {
            w623 = 0.2 ("Delay Time (s)")
            n278 = To Long Integer(number=w604) -> (32bit integer=w636:i32)
            n279 = To Long Integer(number=w601) -> (32bit integer=w637:i32)
            n280 = property on="Y steps/rev" class="DigNum (strict)"() -> ("Value"=w633:u32)  [unwired: 2 in, 2 out]
            n281 = property on="Y offset mm" class="DigNum (strict)"() -> ("Value"=w629:dbl)  [unwired: 2 in, 2 out]
            n282 = To Double Precision Float(number=w633) -> (double precision float=w634:dbl)
            n283 = call "Applied Send Command.vi"("error in (no error)"=w617, "Command"=T1."Immediate Position?", "VISA resource name"=w618) -> ("error out"=w620:errorcluster, "read buffer"=w621:string, "VISA resource name out"=w615:refnum<visa-resource-name>)  [unwired: 4 in]
            n284 = call "Time Delay4"("error in (no error)"=w620, "Delay Time (s)"=w623) -> ("error out"=w613:errorcluster)  [unwired: 9 in]
            n285 = Hexadecimal String To Number(string=w621, offset=3) -> (number=w625:u32)  [unwired: 1 in, 1 out]
            n286 = To Long Integer(number=w625) -> (32bit integer=w627:i32)
            n287 = call "Applied Send Command.vi"("error in (no error)"=w613, "Command"=T1."Request Status", "VISA resource name"=w615) -> ("error out"=w612:errorcluster, "read buffer"=w609:string, "VISA resource name out"=w614:refnum<visa-resource-name>)  [unwired: 4 in]
            n288 = property on="Y Step PV" class="DigNum (strict)"("Val(Sgnl)"=w627) -> ()  [unwired: 2 in, 2 out]
            n289 = call "Time Delay3"("error in (no error)"=w612, "Delay Time (s)"=w623) -> ("error out"=w624:errorcluster)  [unwired: 9 in]
            n290 = String Subset(string=w609, offset (0)=0, length (rest)=1 ("length (rest)")) -> (substring=w607:string)
            n291 = In Range and Coerce(upper limit=w636, x=w627, lower limit=w637) -> (In Range?=w635:bool)  [unwired: 1 out]
            n292 = To Double Precision Float(number=w627) -> (double precision float=w628:dbl)
            n293 = Not Equal?(x=w607, y="R") -> (x != y?=w605:bool)
            n294 = Equal?(x=w607, y="R") -> (x = y?=w622:bool)
            n295 = property on="Y in Motion" class="Bool (strict)"("Val(Sgnl)"=w605) -> ()  [unwired: 2 in, 2 out]
            n296 = property on="Y Ready" class="Bool (strict)"("Val(Sgnl)"=w622) -> ()  [unwired: 2 in, 2 out]
            n297 = Divide(x=w628, y=w634) -> (x/y=w632:dbl)
            n298 = And(x=w635, y=w602) -> (x .and. y?=w603:bool)
            n299 = property on="Y in Range" class="Bool (strict)"("Val(Sgnl)"=w603) -> ()  [unwired: 2 in, 2 out]
            n300 = property on="Y mm/rev" class="DigNum (strict)"() -> ("Value"=w631:dbl)  [unwired: 2 in, 2 out]
            n301 = Multiply(x=w632, y=w631) -> (x*y=w630:dbl)
            n302 = Add(x=w630, y=w629) -> (x+y=w626:dbl)
            n303 = property on="Y Position mm PV" class="DigNum (strict)"("Val(Sgnl)"=w626) -> ()  [unwired: 2 in, 2 out]
          }
          frame #1 {
            n304 = property on="Y Scan" class="Bool (strict)"() -> ("Value"=w640:bool)  [unwired: 2 in, 2 out]
            n305 = Or(x=w639, y=w640) -> (x .or. y?=w641:bool)
            n306 = case shown="True" w641 {
              frame False {
                n307 = property on="Y Scan OK" class="Bool"("DisabledEnum"=T2."Enabled" ("Disabled")) -> ()  [unwired: 2 in, 2 out]
                n308 = property on="Y Go" class="Bool"("DisabledEnum"=T2."Enabled" ("Disabled")) -> ()  [unwired: 2 in, 2 out]
              }
              frame True {
                n309 = property on="Y Scan OK" class="Bool"("DisabledEnum"=T2."Disabled and Grayed Out" ("Disabled")) -> ()  [unwired: 2 in, 2 out]
                n310 = property on="Y Go" class="Bool"("DisabledEnum"=T2."Disabled and Grayed Out" ("Disabled")) -> ()  [unwired: 2 in, 2 out]
              }
            }
          }
          frame #2 {
            n311 = case shown="False" w650 {
              tunnel: w651 -> [w656 w661]
              tunnel: [w658 w661] -> w652
              tunnel: [w657 w660] -> w653
              tunnel: w654 -> [w655 w660]
              frame False {
                n312 = call "Applied Send Command.vi"("error in (no error)"=w655, "Command"=T1."Stop & Kill Buffer", "VISA resource name"=w656) -> ("error out"=w657:errorcluster, "VISA resource name out"=w658:refnum<visa-resource-name>)  [unwired: 4 in, 1 out]
              }
              frame True {
              }
            }
          }
          frame #3 {
            n313 = property on="Y Backlash corr" class="Bool (strict)"() -> ("Value"=w668:bool)  [unwired: 2 in, 2 out]
            n314 = Implies(1:w667, 2:w668) -> (0:w666:bool)
            n315 = case shown="False" w666 {
              tunnel: w665 -> [w671 w700]
              tunnel: w664 -> [w672 w701]
              tunnel: [w669 w700] -> w663
              tunnel: [w670 w701] -> w662
              frame False {
                w678 = 0.1 ("Delay Time (s)")
                # "Backlash"
                n316 = property on="Y Backlash" class="DigNum (strict)"() -> ("Value"=w673:i32)  [unwired: 2 in, 2 out]
                n317 = property on="Y Backlash corr" class="Bool (strict)"("Val(Sgnl)"=FALSE ("Value (Signaling)")) -> ()  [unwired: 2 in, 2 out]
                n318 = To Long Integer(number=w673) -> (32bit integer=w696:i32)
                n319 = Number To Decimal String(number=w673) -> (decimal integer string=w691:string)  [unwired: 1 in]
                n320 = Negate(x=w696) -> (-x=w697:i32)
                n321 = property on="Y Backlash steps/sec" class="DigNum (strict)"() -> ("Value"=w674:i32)  [unwired: 2 in, 2 out]
                n322 = Number To Decimal String(number=w697) -> (decimal integer string=w690:string)  [unwired: 1 in]
                n323 = property on="Y steps/rev" class="DigNum (strict)"() -> ("Value"=w677:u32)  [unwired: 2 in, 2 out]
                n324 = Divide(x=w674, y=w677) -> (x/y=w676:dbl)
                n325 = Number To Fractional String(number=w676) -> (F-format string=w675:string)  [unwired: 3 in]
                n326 = call "Applied Send Command.vi"("error in (no error)"=w671, "Extra"=w675, "Command"=T1."Velocity Setting", "VISA resource name"=w672) -> ("error out"=w680:errorcluster, "VISA resource name out"=w686:refnum<visa-resource-name>)  [unwired: 3 in, 1 out]
                n327 = call "Time Delay41"("error in (no error)"=w680, "Delay Time (s)"=w678) -> ("error out"=w679:errorcluster)  [unwired: 9 in]
                n328 = call "Applied Send Command.vi"("error in (no error)"=w679, "Extra"=w691, "Command"=T1."Distance or Position", "VISA resource name"=w686) -> ("error out"=w685:errorcluster, "VISA resource name out"=w692:refnum<visa-resource-name>)  [unwired: 3 in, 1 out]
                n329 = call "Time Delay38"("error in (no error)"=w685, "Delay Time (s)"=w678) -> ("error out"=w684:errorcluster)  [unwired: 9 in]
                n330 = call "Applied Send Command.vi"("error in (no error)"=w684, "Command"=T1."Feed to Length", "VISA resource name"=w692) -> ("error out"=w683:errorcluster, "VISA resource name out"=w689:refnum<visa-resource-name>)  [unwired: 4 in, 1 out]
                n331 = call "Applied Send Command.vi"("Extra"=w690, "Command"=T1."Distance or Position", "VISA resource name"=w689) -> ("error out"=w682:errorcluster, "VISA resource name out"=w688:refnum<visa-resource-name>)  [unwired: 4 in, 1 out]
                n332 = call "Time Delay39"("error in (no error)"=w683, "Delay Time (s)"=w678) -> ()  [unwired: 9 in, 1 out]
                n333 = call "Time Delay40"("error in (no error)"=w682, "Delay Time (s)"=w678) -> ("error out"=w681:errorcluster)  [unwired: 9 in]
                n334 = call "Applied Send Command.vi"("error in (no error)"=w681, "Command"=T1."Feed to Length", "VISA resource name"=w688) -> ("error out"=w669:errorcluster, "VISA resource name out"=w670:refnum<visa-resource-name>)  [unwired: 4 in, 1 out]
              }
              frame True {
              }
            }
          }
        }
        n335 = Multiply(x=360.0, y=w350) -> (x*y=w353:dbl)
        n336 = property on="atan Y/Z" class="DigNum (strict)"("Val(Sgnl)"=w353) -> ()  [unwired: 2 in, 2 out]
      }
      event "Reset Y Position mm", "Reset X Position mm", "Reset Z Position mm": Value Change {
        n337 = event-data() -> ()  [unwired: 1 in, 5 out]
        n338 = property on="Z steps/rev" class="DigNum (strict)"() -> ("Value"=w704:u32)  [unwired: 2 in, 2 out]
        n339 = property on="X steps/rev" class="DigNum (strict)"() -> ("Value"=w713:u32)  [unwired: 2 in, 2 out]
        n340 = property on="Y steps/rev" class="DigNum (strict)"() -> ("Value"=w722:u32)  [unwired: 2 in, 2 out]
        n341 = property on="Z offset mm" class="DigNum (strict)"() -> ("Value"=w702:dbl)  [unwired: 2 in, 2 out]
        n342 = property on="X offset mm" class="DigNum (strict)"() -> ("Value"=w711:dbl)  [unwired: 2 in, 2 out]
        n343 = property on="Y offset mm" class="DigNum (strict)"() -> ("Value"=w720:dbl)  [unwired: 2 in, 2 out]
        n344 = To Double Precision Float(number=w713) -> (double precision float=w716:dbl)
        n345 = To Double Precision Float(number=w722) -> (double precision float=w725:dbl)
        n346 = property on="Reset Z Position mm" class="DigNum (strict)"() -> ("Value"=w710:dbl)  [unwired: 2 in, 2 out]
        n347 = property on="Reset X Position mm" class="DigNum (strict)"() -> ("Value"=w719:dbl)  [unwired: 2 in, 2 out]
        n348 = property on="Reset Y Position mm" class="DigNum (strict)"() -> ("Value"=w728:dbl)  [unwired: 2 in, 2 out]
        n349 = Subtract(x=w710, y=w702) -> (x-y=w709:dbl)
        n350 = Subtract(x=w719, y=w711) -> (x-y=w718:dbl)
        n351 = Subtract(x=w728, y=w720) -> (x-y=w727:dbl)
        n352 = property on="Z mm/rev" class="DigNum (strict)"() -> ("Value"=w703:dbl)  [unwired: 2 in, 2 out]
        n353 = property on="X mm/rev" class="DigNum (strict)"() -> ("Value"=w712:dbl)  [unwired: 2 in, 2 out]
        n354 = property on="Y mm/rev" class="DigNum (strict)"() -> ("Value"=w721:dbl)  [unwired: 2 in, 2 out]
        n355 = Divide(x=w718, y=w712) -> (x/y=w717:dbl)
        n356 = Divide(x=w727, y=w721) -> (x/y=w726:dbl)
        n357 = Divide(x=w709, y=w703) -> (x/y=w708:dbl)
        n358 = To Double Precision Float(number=w704) -> (double precision float=w707:dbl)
        n359 = Multiply(x=w708, y=w707) -> (x*y=w706:dbl)
        n360 = Multiply(x=w717, y=w716) -> (x*y=w715:dbl)
        n361 = Multiply(x=w726, y=w725) -> (x*y=w724:dbl)
        n362 = To Long Integer(number=w706) -> (32bit integer=w705:i32)
        n363 = To Long Integer(number=w715) -> (32bit integer=w714:i32)
        n364 = To Long Integer(number=w724) -> (32bit integer=w723:i32)
        n365 = property on="Reset Z Motor Steps" class="DigNum (strict)"("Val(Sgnl)"=w705) -> ()  [unwired: 2 in, 2 out]
        n366 = property on="Reset X Motor Steps" class="DigNum (strict)"("Val(Sgnl)"=w714) -> ()  [unwired: 2 in, 2 out]
        n367 = property on="Reset Y Motor Steps" class="DigNum (strict)"("Val(Sgnl)"=w723) -> ()  [unwired: 2 in, 2 out]
      }
      event "Y Velocity SP step/sec", "X Velocity SP step/sec", "Z Velocity SP step/sec", "Y Step SP", "X Step SP", "Z Step SP": Value Change {
        n368 = event-data() -> ()  [unwired: 1 in, 5 out]
        n369 = property on="Z Step SP" class="DigNum (strict)"() -> ("Value"=w735:i32)  [unwired: 2 in, 2 out]
        n370 = property on="Y Step SP" class="DigNum (strict)"() -> ("Value"=w751:i32)  [unwired: 2 in, 2 out]
        n371 = property on="X Step SP" class="DigNum (strict)"() -> ("Value"=w743:i32)  [unwired: 2 in, 2 out]
        n372 = property on="Z steps/rev" class="DigNum (strict)"() -> ("Value"=w756:u32)  [unwired: 2 in, 2 out]
        n373 = property on="Z steps/rev" class="DigNum (strict)"() -> ("Value"=w733:u32)  [unwired: 2 in, 2 out]
        n374 = property on="Y steps/rev" class="DigNum (strict)"() -> ("Value"=w768:u32)  [unwired: 2 in, 2 out]
        n375 = property on="Y steps/rev" class="DigNum (strict)"() -> ("Value"=w749:u32)  [unwired: 2 in, 2 out]
        n376 = property on="X steps/rev" class="DigNum (strict)"() -> ("Value"=w762:u32)  [unwired: 2 in, 2 out]
        n377 = property on="X steps/rev" class="DigNum (strict)"() -> ("Value"=w741:u32)  [unwired: 2 in, 2 out]
        n378 = property on="Z offset mm" class="DigNum (strict)"() -> ("Value"=w732:dbl)  [unwired: 2 in, 2 out]
        n379 = property on="Y offset mm" class="DigNum (strict)"() -> ("Value"=w748:dbl)  [unwired: 2 in, 2 out]
        n380 = property on="X offset mm" class="DigNum (strict)"() -> ("Value"=w740:dbl)  [unwired: 2 in, 2 out]
        n381 = To Double Precision Float(number=w756) -> (double precision float=w761:dbl)
        n382 = To Double Precision Float(number=w735) -> (double precision float=w736:dbl)
        n383 = To Double Precision Float(number=w733) -> (double precision float=w739:dbl)
        n384 = To Double Precision Float(number=w751) -> (double precision float=w752:dbl)
        n385 = To Double Precision Float(number=w749) -> (double precision float=w755:dbl)
        n386 = To Double Precision Float(number=w762) -> (double precision float=w767:dbl)
        n387 = To Double Precision Float(number=w743) -> (double precision float=w744:dbl)
        n388 = To Double Precision Float(number=w741) -> (double precision float=w747:dbl)
        n389 = Divide(x=w736, y=w739) -> (x/y=w738:dbl)
        n390 = Divide(x=w752, y=w755) -> (x/y=w754:dbl)
        n391 = Divide(x=w744, y=w747) -> (x/y=w746:dbl)
        n392 = property on="Z Velocity SP step/sec" class="DigNum (strict)"() -> ("Value"=w758:i32)  [unwired: 2 in, 2 out]
        n393 = property on="Z mm/rev" class="DigNum (strict)"() -> ("Value"=w731:dbl)  [unwired: 2 in, 2 out]
        n394 = property on="Y Velocity SP step/sec" class="DigNum (strict)"() -> ("Value"=w770:i32)  [unwired: 2 in, 2 out]
        n395 = property on="Y mm/rev" class="DigNum (strict)"() -> ("Value"=w729:dbl)  [unwired: 2 in, 2 out]
        n396 = property on="X Velocity SP step/sec" class="DigNum (strict)"() -> ("Value"=w764:i32)  [unwired: 2 in, 2 out]
        n397 = property on="X mm/rev" class="DigNum (strict)"() -> ("Value"=w730:dbl)  [unwired: 2 in, 2 out]
        n398 = Multiply(x=w738, y=w731) -> (x*y=w737:dbl)
        n399 = Multiply(x=w754, y=w729) -> (x*y=w753:dbl)
        n400 = Multiply(x=w746, y=w730) -> (x*y=w745:dbl)
        n401 = To Double Precision Float(number=w758) -> (double precision float=w759:dbl)
        n402 = To Double Precision Float(number=w770) -> (double precision float=w771:dbl)
        n403 = To Double Precision Float(number=w768) -> (double precision float=w773:dbl)
        n404 = To Double Precision Float(number=w764) -> (double precision float=w765:dbl)
        n405 = Divide(x=w759, y=w761) -> (x/y=w760:dbl)
        n406 = Add(x=w737, y=w732) -> (x+y=w734:dbl)
        n407 = Divide(x=w771, y=w773) -> (x/y=w772:dbl)
        n408 = Add(x=w753, y=w748) -> (x+y=w750:dbl)
        n409 = Divide(x=w765, y=w767) -> (x/y=w766:dbl)
        n410 = Add(x=w745, y=w740) -> (x+y=w742:dbl)
        n411 = Multiply(x=w760, y=w731) -> (x*y=w757:dbl)
        n412 = property on="Z Position MV mm" class="DigNum (strict)"("Val(Sgnl)"=w734) -> ()  [unwired: 2 in, 2 out]
        n413 = Multiply(x=w772, y=w729) -> (x*y=w769:dbl)
        n414 = property on="Y Position MV mm" class="DigNum (strict)"("Val(Sgnl)"=w750) -> ()  [unwired: 2 in, 2 out]
        n415 = Multiply(x=w766, y=w730) -> (x*y=w763:dbl)
        n416 = property on="X Position MV mm" class="DigNum (strict)"("Val(Sgnl)"=w742) -> ()  [unwired: 2 in, 2 out]
        n417 = property on="Z Velocity MV mm/sec" class="DigNum (strict)"("Val(Sgnl)"=w757) -> ()  [unwired: 2 in, 2 out]
        n418 = property on="Y Velocity MV mm/sec" class="DigNum (strict)"("Val(Sgnl)"=w769) -> ()  [unwired: 2 in, 2 out]
        n419 = property on="X Velocity MV mm/sec" class="DigNum (strict)"("Val(Sgnl)"=w763) -> ()  [unwired: 2 in, 2 out]
      }
      event "Y Scan Length SP steps", "Y Scan Velocity SP steps/sec", "X Scan Velocity SP steps/sec", "X Scan Length SP steps", "Z Scan Velocity SP steps/sec", "Z Scan Length SP steps": Value Change {
        n420 = event-data() -> ()  [unwired: 1 in, 5 out]
        n421 = property on="Z steps/rev" class="DigNum (strict)"() -> ("Value"=w797:u32)  [unwired: 2 in, 2 out]
        n422 = property on="X steps/rev" class="DigNum (strict)"() -> ("Value"=w824:u32)  [unwired: 2 in, 2 out]
        n423 = property on="Y steps/rev" class="DigNum (strict)"() -> ("Value"=w810:u32)  [unwired: 2 in, 2 out]
        n424 = property on="X Step PV" class="DigNum (strict)"() -> ("Value"=w822:i32)  [unwired: 2 in, 2 out]
        n425 = property on="Y Step PV" class="DigNum (strict)"() -> ("Value"=w808:i32)  [unwired: 2 in, 2 out]
        n426 = property on="Z Step PV" class="DigNum (strict)"() -> ("Value"=w795:i32)  [unwired: 2 in, 2 out]
        n427 = To Double Precision Float(number=w822) -> (double precision float=w789:dbl)
        n428 = To Double Precision Float(number=w808) -> (double precision float=w788:dbl)
        n429 = To Double Precision Float(number=w795) -> (double precision float=w787:dbl)
        n430 = To Double Precision Float(number=w797) -> (double precision float=w794:dbl)
        n431 = To Double Precision Float(number=w824) -> (double precision float=w821:dbl)
        n432 = To Double Precision Float(number=w810) -> (double precision float=w783:dbl)
        n433 = property on="X Step SP" class="DigNum (strict)"() -> ("Maximum"=w828:dbl)  [unwired: 2 in, 2 out]
        n434 = property on="Y Step SP" class="DigNum (strict)"() -> ("Maximum"=w814:dbl)  [unwired: 2 in, 2 out]
        n435 = property on="Z Step SP" class="DigNum (strict)"() -> ("Maximum"=w801:dbl)  [unwired: 2 in, 2 out]
        n436 = property on="X Step SP" class="DigNum (strict)"() -> ("Minimum"=w829:dbl)  [unwired: 2 in, 2 out]
        n437 = property on="Y Step SP" class="DigNum (strict)"() -> ("Minimum"=w815:dbl)  [unwired: 2 in, 2 out]
        n438 = property on="Z Step SP" class="DigNum (strict)"() -> ("Minimum"=w802:dbl)  [unwired: 2 in, 2 out]
        n439 = property on="Z Scan Length SP steps" class="DigNum (strict)"() -> ("Value"=w798:i32)  [unwired: 2 in, 2 out]
        n440 = property on="X Scan Length SP steps" class="DigNum (strict)"() -> ("Value"=w820:i32)  [unwired: 2 in, 2 out]
        n441 = property on="Y Scan Length SP steps" class="DigNum (strict)"() -> ("Value"=w811:i32)  [unwired: 2 in, 2 out]
        n442 = property on="Z Scan Velocity SP steps/sec" class="DigNum (strict)"() -> ("Value"=w793:i32)  [unwired: 2 in, 2 out]
        n443 = property on="X Scan Velocity SP steps/sec" class="DigNum (strict)"() -> ("Value"=w825:i32)  [unwired: 2 in, 2 out]
        n444 = property on="Y Scan Velocity SP steps/sec" class="DigNum (strict)"() -> ("Value"=w807:i32)  [unwired: 2 in, 2 out]
        n445 = Subtract(x=w829, y=w789) -> (x-y=w830:dbl)
        n446 = Subtract(x=w828, y=w789) -> (x-y=w827:dbl)
        n447 = Subtract(x=w815, y=w788) -> (x-y=w816:dbl)
        n448 = Subtract(x=w814, y=w788) -> (x-y=w813:dbl)
        n449 = Subtract(x=w802, y=w787) -> (x-y=w803:dbl)
        n450 = Subtract(x=w801, y=w787) -> (x-y=w800:dbl)
        n451 = To Double Precision Float(number=w798) -> (double precision float=w786:dbl)
        n452 = To Double Precision Float(number=w820) -> (double precision float=w778:dbl)
        n453 = To Double Precision Float(number=w811) -> (double precision float=w782:dbl)
        n454 = property on="X Scan Length SP steps" class="DigNum (strict)"("Minimum"=w830) -> ()  [unwired: 2 in, 2 out]
        n455 = property on="Y Scan Length SP steps" class="DigNum (strict)"("Minimum"=w816) -> ()  [unwired: 2 in, 2 out]
        n456 = property on="Z Scan Length SP steps" class="DigNum (strict)"("Minimum"=w803) -> ()  [unwired: 2 in, 2 out]
        n457 = property on="X Scan Length SP steps" class="DigNum (strict)"("Maximum"=w827) -> ()  [unwired: 2 in, 2 out]
        n458 = property on="Y Scan Length SP steps" class="DigNum (strict)"("Maximum"=w813) -> ()  [unwired: 2 in, 2 out]
        n459 = property on="Z Scan Length SP steps" class="DigNum (strict)"("Maximum"=w800) -> ()  [unwired: 2 in, 2 out]
        n460 = Divide(x=w786, y=w794) -> (x/y=w799:dbl)
        n461 = Divide(x=w778, y=w821) -> (x/y=w819:dbl)
        n462 = Divide(x=w782, y=w783) -> (x/y=w812:dbl)
        n463 = To Double Precision Float(number=w793) -> (double precision float=w785:dbl)
        n464 = To Double Precision Float(number=w825) -> (double precision float=w777:dbl)
        n465 = To Double Precision Float(number=w807) -> (double precision float=w781:dbl)
        n466 = property on="Z mm/rev" class="DigNum (strict)"() -> ("Value"=w796:dbl)  [unwired: 2 in, 2 out]
        n467 = property on="X mm/rev" class="DigNum (strict)"() -> ("Value"=w823:dbl)  [unwired: 2 in, 2 out]
        n468 = property on="Y mm/rev" class="DigNum (strict)"() -> ("Value"=w809:dbl)  [unwired: 2 in, 2 out]
        n469 = Multiply(x=w799, y=w796) -> (x*y=w791:dbl)
        n470 = Divide(x=w786, y=w785) -> (x/y=w784:dbl)
        n471 = Divide(x=w785, y=w794) -> (x/y=w792:dbl)
        n472 = Multiply(x=w823, y=w819) -> (x*y=w817:dbl)
        n473 = Divide(x=w778, y=w777) -> (x/y=w779:dbl)
        n474 = Divide(x=w777, y=w821) -> (x/y=w826:dbl)
        n475 = Multiply(x=w812, y=w809) -> (x*y=w805:dbl)
        n476 = Divide(x=w782, y=w781) -> (x/y=w780:dbl)
        n477 = Divide(x=w781, y=w783) -> (x/y=w806:dbl)
        n478 = Multiply(x=w796, y=w792) -> (x*y=w790:dbl)
        n479 = property on="X Scan length MV mm" class="DigNum (strict)"("Val(Sgnl)"=w817) -> ()  [unwired: 2 in, 2 out]
        n480 = Multiply(x=w826, y=w823) -> (x*y=w818:dbl)
        n481 = Multiply(x=w809, y=w806) -> (x*y=w804:dbl)
        n482 = property on="Z Scan length MV mm" class="DigNum (strict)"("Value"=w791) -> ()  [unwired: 2 in, 2 out]
        n483 = Absolute Value(x=w784) -> (abs(x)=→"Z Scan Duration":dbl)
        n484 = Absolute Value(x=w779) -> (abs(x)=→"X Scan Duration":dbl)
        n485 = property on="Y Scan length MV mm" class="DigNum (strict)"("Value"=w805) -> ()  [unwired: 2 in, 2 out]
        n486 = Absolute Value(x=w780) -> (abs(x)=→"Y Scan Duration":dbl)
        n487 = property on="Z Scan velocity MV mm/sec" class="DigNum (strict)"("Val(Sgnl)"=w790) -> ()  [unwired: 2 in, 2 out]
        n488 = property on="Y Scan velocity MV mm/sec" class="DigNum (strict)"("Val(Sgnl)"=w804) -> ()  [unwired: 2 in, 2 out]
        n489 = property on="X Scan velocity MV mm/sec" class="DigNum (strict)"("Value"=w818) -> ()  [unwired: 2 in, 2 out]
      }
      event "Y Move Set": Mouse Down {
        n490 = event-data() -> ()  [unwired: 1 in, 7 out]
        n491 = property on="Y steps/rev" class="DigNum (strict)"() -> ("Value"=w847:u32)  [unwired: 2 in, 2 out]
        n492 = property on="Y offset mm" class="DigNum (strict)"() -> ("Value"=w845:dbl)  [unwired: 2 in, 2 out]
        n493 = property on="Y Position SP mm" class="DigNum (strict)"() -> ("Value"=w844:dbl)  [unwired: 2 in, 2 out]
        n494 = property on="Y Velocity SP step/sec" class="DigNum (strict)"() -> ("Maximum"=w834:dbl)  [unwired: 2 in, 2 out]
        n495 = property on="Y Velocity SP step/sec" class="DigNum (strict)"() -> ("Minimum"=w833:dbl)  [unwired: 2 in, 2 out]
        n496 = Subtract(x=w844, y=w845) -> (x-y=w848:dbl)
        n497 = property on="Y Velocity SP mm/sec" class="DigNum (strict)"() -> ("Value"=w838:dbl)  [unwired: 2 in, 2 out]
        n498 = property on="Y mm/rev" class="DigNum (strict)"() -> ("Value"=w831:dbl)  [unwired: 2 in, 2 out]
        n499 = Divide(x=w848, y=w831) -> (x/y=w849:dbl)
        n500 = Divide(x=w838, y=w831) -> (x/y=w839:dbl)
        n501 = To Double Precision Float(number=w847) -> (double precision float=w832:dbl)
        n502 = Multiply(x=w849, y=w832) -> (x*y=w843:dbl)
        n503 = Multiply(x=w839, y=w832) -> (x*y=w836:dbl)
        n504 = property on="Y Step SP" class="DigNum (strict)"() -> ("Maximum"=w841:dbl)  [unwired: 2 in, 2 out]
        n505 = property on="Y Step SP" class="DigNum (strict)"() -> ("Minimum"=w840:dbl)  [unwired: 2 in, 2 out]
        n506 = In Range and Coerce(upper limit=w834, x=w836, lower limit=w833) -> (coerced(x)=w835:dbl)  [unwired: 1 out]
        n507 = To Long Integer(number=w835) -> (32bit integer=w837:i32)
        n508 = In Range and Coerce(upper limit=w841, x=w843, lower limit=w840) -> (coerced(x)=w842:dbl)  [unwired: 1 out]
        n509 = property on="Y Velocity SP step/sec" class="DigNum (strict)"("Val(Sgnl)"=w837) -> ()  [unwired: 2 in, 2 out]
        n510 = To Long Integer(number=w842) -> (32bit integer=w846:i32)
        n511 = property on="Y Step SP" class="DigNum (strict)"("Val(Sgnl)"=w846) -> ()  [unwired: 2 in, 2 out]
      }
      event "X Move Set": Mouse Down {
        n512 = event-data() -> ()  [unwired: 1 in, 7 out]
        n513 = property on="X steps/rev" class="DigNum (strict)"() -> ("Value"=w866:u32)  [unwired: 2 in, 2 out]
        n514 = property on="X offset mm" class="DigNum (strict)"() -> ("Value"=w864:dbl)  [unwired: 2 in, 2 out]
        n515 = property on="X Position SP mm" class="DigNum (strict)"() -> ("Value"=w863:dbl)  [unwired: 2 in, 2 out]
        n516 = property on="X Velocity SP step/sec" class="DigNum (strict)"() -> ("Maximum"=w853:dbl)  [unwired: 2 in, 2 out]
        n517 = property on="X Velocity SP step/sec" class="DigNum (strict)"() -> ("Minimum"=w852:dbl)  [unwired: 2 in, 2 out]
        n518 = Subtract(x=w863, y=w864) -> (x-y=w867:dbl)
        n519 = property on="X Velocity SP mm/sec" class="DigNum (strict)"() -> ("Value"=w857:dbl)  [unwired: 2 in, 2 out]
        n520 = property on="X mm/rev" class="DigNum (strict)"() -> ("Value"=w850:dbl)  [unwired: 2 in, 2 out]
        n521 = Divide(x=w867, y=w850) -> (x/y=w868:dbl)
        n522 = Divide(x=w857, y=w850) -> (x/y=w858:dbl)
        n523 = To Double Precision Float(number=w866) -> (double precision float=w851:dbl)
        n524 = Multiply(x=w868, y=w851) -> (x*y=w862:dbl)
        n525 = Multiply(x=w858, y=w851) -> (x*y=w855:dbl)
        n526 = property on="X Step SP" class="DigNum (strict)"() -> ("Maximum"=w860:dbl)  [unwired: 2 in, 2 out]
        n527 = property on="X Step SP" class="DigNum (strict)"() -> ("Minimum"=w859:dbl)  [unwired: 2 in, 2 out]
        n528 = In Range and Coerce(upper limit=w853, x=w855, lower limit=w852) -> (coerced(x)=w854:dbl)  [unwired: 1 out]
        n529 = To Long Integer(number=w854) -> (32bit integer=w856:i32)
        n530 = In Range and Coerce(upper limit=w860, x=w862, lower limit=w859) -> (coerced(x)=w861:dbl)  [unwired: 1 out]
        n531 = property on="X Velocity SP step/sec" class="DigNum (strict)"("Val(Sgnl)"=w856) -> ()  [unwired: 2 in, 2 out]
        n532 = To Long Integer(number=w861) -> (32bit integer=w865:i32)
        n533 = property on="X Step SP" class="DigNum (strict)"("Val(Sgnl)"=w865) -> ()  [unwired: 2 in, 2 out]
      }
      event "Z Move Set": Mouse Down {
        n534 = event-data() -> ()  [unwired: 1 in, 7 out]
        n535 = property on="Z steps/rev" class="DigNum (strict)"() -> ("Value"=w883:u32)  [unwired: 2 in, 2 out]
        n536 = property on="Z offset mm" class="DigNum (strict)"() -> ("Value"=w881:dbl)  [unwired: 2 in, 2 out]
        n537 = property on="Z Position SP mm" class="DigNum (strict)"() -> ("Value"=w880:dbl)  [unwired: 2 in, 2 out]
        n538 = property on="Z Velocity SP step/sec" class="DigNum (strict)"() -> ("Maximum"=w870:dbl)  [unwired: 2 in, 2 out]
        n539 = property on="Z Velocity SP step/sec" class="DigNum (strict)"() -> ("Minimum"=w869:dbl)  [unwired: 2 in, 2 out]
        n540 = Subtract(x=w880, y=w881) -> (x-y=w884:dbl)
        n541 = property on="Z Velocity SP mm/sec" class="DigNum (strict)"() -> ("Value"=w874:dbl)  [unwired: 2 in, 2 out]
        n542 = property on="Z mm/rev" class="DigNum (strict)"() -> ("Value"=w886:dbl)  [unwired: 2 in, 2 out]
        n543 = Divide(x=w884, y=w886) -> (x/y=w885:dbl)
        n544 = Divide(x=w874, y=w886) -> (x/y=w875:dbl)
        n545 = To Double Precision Float(number=w883) -> (double precision float=w887:dbl)
        n546 = Multiply(x=w885, y=w887) -> (x*y=w879:dbl)
        n547 = Multiply(x=w875, y=w887) -> (x*y=w872:dbl)
        n548 = property on="Z Step SP" class="DigNum (strict)"() -> ("Maximum"=w877:dbl)  [unwired: 2 in, 2 out]
        n549 = property on="Z Step SP" class="DigNum (strict)"() -> ("Minimum"=w876:dbl)  [unwired: 2 in, 2 out]
        n550 = In Range and Coerce(upper limit=w870, x=w872, lower limit=w869) -> (coerced(x)=w871:dbl)  [unwired: 1 out]
        n551 = To Long Integer(number=w871) -> (32bit integer=w873:i32)
        n552 = In Range and Coerce(upper limit=w877, x=w879, lower limit=w876) -> (coerced(x)=w878:dbl)  [unwired: 1 out]
        n553 = property on="Z Velocity SP step/sec" class="DigNum (strict)"("Val(Sgnl)"=w873) -> ()  [unwired: 2 in, 2 out]
        n554 = To Long Integer(number=w878) -> (32bit integer=w882:i32)
        n555 = property on="Z Step SP" class="DigNum (strict)"("Val(Sgnl)"=w882) -> ()  [unwired: 2 in, 2 out]
      }
      event "Y Scan set": Mouse Down {
        n556 = event-data() -> ()  [unwired: 1 in, 7 out]
        n557 = property on="Y steps/rev" class="DigNum (strict)"() -> ("Value"=w903:u32)  [unwired: 2 in, 2 out]
        n558 = To Double Precision Float(number=w903) -> (double precision float=w889:dbl)
        n559 = property on="Y mm/rev" class="DigNum (strict)"() -> ("Value"=w888:dbl)  [unwired: 2 in, 2 out]
        n560 = property on="Y Scan Length SP mm" class="DigNum (strict)"() -> ("Value"=w901:dbl)  [unwired: 2 in, 2 out]
        n561 = property on="Y Scan Velocity SP mm/sec" class="DigNum (strict)"() -> ("Value"=w895:dbl)  [unwired: 2 in, 2 out]
        n562 = property on="Y Scan Velocity SP steps/sec" class="DigNum (strict)"() -> ("Maximum"=w891:dbl)  [unwired: 2 in, 2 out]
        n563 = property on="Y Scan Velocity SP steps/sec" class="DigNum (strict)"() -> ("Minimum"=w890:dbl)  [unwired: 2 in, 2 out]
        n564 = Divide(x=w901, y=w888) -> (x/y=w904:dbl)
        n565 = Divide(x=w895, y=w888) -> (x/y=w896:dbl)
        n566 = Multiply(x=w904, y=w889) -> (x*y=w900:dbl)
        n567 = Multiply(x=w896, y=w889) -> (x*y=w893:dbl)
        n568 = property on="Y Step SP" class="DigNum (strict)"() -> ("Maximum"=w897:dbl)  [unwired: 2 in, 2 out]
        n569 = property on="Y Step SP" class="DigNum (strict)"() -> ("Minimum"=w898:dbl)  [unwired: 2 in, 2 out]
        n570 = In Range and Coerce(upper limit=w891, x=w893, lower limit=w890) -> (coerced(x)=w892:dbl)  [unwired: 1 out]
        n571 = To Long Integer(number=w892) -> (32bit integer=w894:i32)
        n572 = In Range and Coerce(upper limit=w897, x=w900, lower limit=w898) -> (coerced(x)=w899:dbl)  [unwired: 1 out]
        n573 = property on="Y Scan Velocity SP steps/sec" class="DigNum (strict)"("Val(Sgnl)"=w894) -> ()  [unwired: 2 in, 2 out]
        n574 = To Long Integer(number=w899) -> (32bit integer=w902:i32)
        n575 = property on="Y Scan Length SP steps" class="DigNum (strict)"("Val(Sgnl)"=w902) -> ()  [unwired: 2 in, 2 out]
      }
      event "X Scan set": Mouse Down {
        n576 = event-data() -> ()  [unwired: 1 in, 7 out]
        n577 = property on="X steps/rev" class="DigNum (strict)"() -> ("Value"=w920:u32)  [unwired: 2 in, 2 out]
        n578 = To Double Precision Float(number=w920) -> (double precision float=w906:dbl)
        n579 = property on="X mm/rev" class="DigNum (strict)"() -> ("Value"=w905:dbl)  [unwired: 2 in, 2 out]
        n580 = property on="X Scan Length SP mm" class="DigNum (strict)"() -> ("Value"=w918:dbl)  [unwired: 2 in, 2 out]
        n581 = property on="X Scan Velocity SP mm/sec" class="DigNum (strict)"() -> ("Value"=w912:dbl)  [unwired: 2 in, 2 out]
        n582 = property on="X Scan Velocity SP steps/sec" class="DigNum (strict)"() -> ("Maximum"=w908:dbl)  [unwired: 2 in, 2 out]
        n583 = property on="X Scan Velocity SP steps/sec" class="DigNum (strict)"() -> ("Minimum"=w907:dbl)  [unwired: 2 in, 2 out]
        n584 = Divide(x=w918, y=w905) -> (x/y=w921:dbl)
        n585 = Divide(x=w912, y=w905) -> (x/y=w913:dbl)
        n586 = Multiply(x=w921, y=w906) -> (x*y=w917:dbl)
        n587 = Multiply(x=w913, y=w906) -> (x*y=w910:dbl)
        n588 = property on="X Step SP" class="DigNum (strict)"() -> ("Maximum"=w914:dbl)  [unwired: 2 in, 2 out]
        n589 = property on="X Step SP" class="DigNum (strict)"() -> ("Minimum"=w915:dbl)  [unwired: 2 in, 2 out]
        n590 = In Range and Coerce(upper limit=w908, x=w910, lower limit=w907) -> (coerced(x)=w909:dbl)  [unwired: 1 out]
        n591 = To Long Integer(number=w909) -> (32bit integer=w911:i32)
        n592 = In Range and Coerce(upper limit=w914, x=w917, lower limit=w915) -> (coerced(x)=w916:dbl)  [unwired: 1 out]
        n593 = property on="X Scan Velocity SP steps/sec" class="DigNum (strict)"("Val(Sgnl)"=w911) -> ()  [unwired: 2 in, 2 out]
        n594 = To Long Integer(number=w916) -> (32bit integer=w919:i32)
        n595 = property on="X Scan Length SP steps" class="DigNum (strict)"("Val(Sgnl)"=w919) -> ()  [unwired: 2 in, 2 out]
      }
      event "Z Scan set": Mouse Down {
        n596 = event-data() -> ()  [unwired: 1 in, 7 out]
        n597 = property on="Z steps/rev" class="DigNum (strict)"() -> ("Value"=w937:u32)  [unwired: 2 in, 2 out]
        n598 = To Double Precision Float(number=w937) -> (double precision float=w923:dbl)
        n599 = property on="Z mm/rev" class="DigNum (strict)"() -> ("Value"=w922:dbl)  [unwired: 2 in, 2 out]
        n600 = property on="Z Scan Length SP mm" class="DigNum (strict)"() -> ("Value"=w935:dbl)  [unwired: 2 in, 2 out]
        n601 = property on="Z Scan Velocity SP mm/sec" class="DigNum (strict)"() -> ("Value"=w929:dbl)  [unwired: 2 in, 2 out]
        n602 = property on="Z Scan Velocity SP steps/sec" class="DigNum (strict)"() -> ("Maximum"=w925:dbl)  [unwired: 2 in, 2 out]
        n603 = property on="Z Scan Velocity SP steps/sec" class="DigNum (strict)"() -> ("Minimum"=w924:dbl)  [unwired: 2 in, 2 out]
        n604 = Divide(x=w935, y=w922) -> (x/y=w938:dbl)
        n605 = Divide(x=w929, y=w922) -> (x/y=w930:dbl)
        n606 = Multiply(x=w938, y=w923) -> (x*y=w934:dbl)
        n607 = Multiply(x=w930, y=w923) -> (x*y=w927:dbl)
        n608 = property on="Z Step SP" class="DigNum (strict)"() -> ("Maximum"=w931:dbl)  [unwired: 2 in, 2 out]
        n609 = property on="Z Step SP" class="DigNum (strict)"() -> ("Minimum"=w932:dbl)  [unwired: 2 in, 2 out]
        n610 = In Range and Coerce(upper limit=w925, x=w927, lower limit=w924) -> (coerced(x)=w926:dbl)  [unwired: 1 out]
        n611 = To Long Integer(number=w926) -> (32bit integer=w928:i32)
        n612 = In Range and Coerce(upper limit=w931, x=w934, lower limit=w932) -> (coerced(x)=w933:dbl)  [unwired: 1 out]
        n613 = property on="Z Scan Velocity SP steps/sec" class="DigNum (strict)"("Val(Sgnl)"=w928) -> ()  [unwired: 2 in, 2 out]
        n614 = To Long Integer(number=w933) -> (32bit integer=w936:i32)
        n615 = property on="Z Scan Length SP steps" class="DigNum (strict)"("Val(Sgnl)"=w936) -> ()  [unwired: 2 in, 2 out]
      }
      event "Y Go": Mouse Up {
        n616 = event-data() -> ()  [unwired: 1 in, 7 out]
        n617 = flat-sequence {
          tunnel: w945 -> [w955]
          tunnel: w946 -> [w956]
          tunnel: [w956] -> w942
          tunnel: [w955] -> w941
          tunnel: [w959] -> w944
          tunnel: [w958] -> w943
          tunnel: w942 -> [w961]
          tunnel: w941 -> [w960]
          tunnel: [w982] -> w948
          tunnel: [w977] -> w947
          tunnel: w944 -> [w981]
          tunnel: w943 -> [w980]
          tunnel: [w976] -> w940
          tunnel: [w993] -> w950
          tunnel: [w988] -> w949
          tunnel: w948 -> [w991]
          tunnel: w947 -> [w992]
          tunnel: w940 -> [w989]
          tunnel: [w989] -> w939
          tunnel: [w996] -> w951
          tunnel: [w999] -> w952
          tunnel: w950 -> [w998]
          tunnel: w949 -> [w997]
          tunnel: w939 -> [w1000]
          frame #0 {
            n618 = property on="Scan Go" class="Bool"("DisabledEnum"=T2."Disabled and Grayed Out" ("Disabled")) -> ()  [unwired: 2 in, 2 out]
            n619 = property on="Y Go" class="Bool"("DisabledEnum"=T2."Disabled and Grayed Out" ("Disabled")) -> ()  [unwired: 2 in, 2 out]
          }
          frame #1 {
            n620 = property on="Y Step SP" class="DigNum (strict)"() -> ("Value"=w969:i32)  [unwired: 2 in, 2 out]
            n621 = property on="Y Step PV" class="DigNum (strict)"() -> ("Value"=w968:i32)  [unwired: 2 in, 2 out]
            n622 = property on="Y Backlash" class="DigNum (strict)"() -> ("Value"=w957:i32)  [unwired: 2 in, 2 out]
            n623 = Subtract(x=w969, y=w968) -> (x-y=w967:i32)
            n624 = Sign(1:w957) -> (0:w965:i32)
            n625 = Sign(1:w967) -> (0:w966:i32)
            n626 = Multiply(x=w966, y=w965) -> (x*y=w964:i32)
            n627 = Equal?(x=w964, y=1) -> (x = y?=w962:bool)
            n628 = case shown="False" w962 {
              tunnel: w961 -> [w972 w974]
              tunnel: w960 -> [w971 w973]
              tunnel: [w971 w973] -> w959
              tunnel: [w972 w974] -> w958
              frame False {
                n629 = property on="Y Backlash corr" class="Bool (strict)"("Val(Sgnl)"=FALSE ("Value (Signaling)")) -> ()  [unwired: 2 in, 2 out]
              }
              frame True {
                n630 = property on="Y Backlash corr" class="Bool (strict)"("Val(Sgnl)"=TRUE ("Value (Signaling)")) -> ()  [unwired: 2 in, 2 out]
              }
            }
          }
          frame #2 {
            w976 = 0.1 ("Delay Time (s)")
            # "Velocity Setting"
            n631 = property on="Y Velocity SP step/sec" class="DigNum (strict)"() -> ("Value"=w985:i32)  [unwired: 2 in, 2 out]
            n632 = Number To Decimal String(number=w985) -> ()  [unwired: 1 in, 1 out]
            n633 = property on="Y steps/rev" class="DigNum (strict)"() -> ("Value"=w984:u32)  [unwired: 2 in, 2 out]
            n634 = Divide(x=w985, y=w984) -> (x/y=w986:dbl)
            n635 = Number To Fractional String(number=w986) -> (F-format string=w979:string)  [unwired: 3 in]
            n636 = call "Applied Send Command.vi"("error in (no error)"=w981, "Extra"=w979, "Command"=T1."Velocity Setting", "VISA resource name"=w980) -> ("error out"=w978:errorcluster, "VISA resource name out"=w982:refnum<visa-resource-name>)  [unwired: 3 in, 1 out]
            n637 = call "Time Delay22"("error in (no error)"=w978, "Delay Time (s)"=w976) -> ("error out"=w977:errorcluster)  [unwired: 9 in]
          }
          frame #3 {
            # "Move to Abs Position"
            n638 = property on="Y Step SP" class="DigNum (strict)"() -> ("Value"=w995:i32)  [unwired: 2 in, 2 out]
            n639 = Number To Decimal String(number=w995) -> (decimal integer string=w990:string)  [unwired: 1 in]
            n640 = call "Applied Send Command.vi"("error in (no error)"=w992, "Extra"=w990, "Command"=T1."Distance or Position", "VISA resource name"=w991) -> ("error out"=w987:errorcluster, "VISA resource name out"=w993:refnum<visa-resource-name>)  [unwired: 3 in, 1 out]
            n641 = call "Time Delay"("error in (no error)"=w987, "Delay Time (s)"=w989) -> ("error out"=w988:errorcluster)  [unwired: 9 in]
          }
          frame #4 {
            n642 = call "Applied Send Command.vi"("error in (no error)"=w997, "Command"=T1."Feed to Position", "VISA resource name"=w998) -> ("error out"=w1001:errorcluster, "VISA resource name out"=w999:refnum<visa-resource-name>)  [unwired: 4 in, 1 out]
            n643 = call "Time Delay23"("error in (no error)"=w1001, "Delay Time (s)"=w1000) -> ("error out"=w996:errorcluster)  [unwired: 9 in]
          }
        }
      }
      event "Z Go": Mouse Up {
        n644 = event-data() -> ()  [unwired: 1 in, 7 out]
        n645 = flat-sequence {
          tunnel: w1007 -> [w1019]
          tunnel: w1008 -> [w1020]
          tunnel: [w1020] -> w1010
          tunnel: [w1019] -> w1009
          tunnel: [w1023] -> w1012
          tunnel: [w1022] -> w1011
          tunnel: w1010 -> [w1025]
          tunnel: w1009 -> [w1024]
          tunnel: [w1043] -> w1014
          tunnel: [w1041] -> w1013
          tunnel: w1012 -> [w1044]
          tunnel: w1011 -> [w1045]
          tunnel: [w1040] -> w1004
          tunnel: [w1054] -> w1016
          tunnel: [w1053] -> w1015
          tunnel: w1014 -> [w1055]
          tunnel: w1013 -> [w1057]
          tunnel: w1004 -> [w1051]
          tunnel: [w1051] -> w1003
          tunnel: [w1066] -> w1006
          tunnel: [w1062] -> w1005
          tunnel: w1016 -> [w1063]
          tunnel: w1015 -> [w1060]
          tunnel: w1003 -> [w1065]
          frame #0 {
            n646 = property on="Scan Go" class="Bool"("DisabledEnum"=T2."Disabled and Grayed Out" ("Disabled")) -> ()  [unwired: 2 in, 2 out]
            n647 = property on="Z Go" class="Bool"("DisabledEnum"=T2."Disabled and Grayed Out" ("Disabled")) -> ()  [unwired: 2 in, 2 out]
          }
          frame #1 {
            n648 = property on="Z Step SP" class="DigNum (strict)"() -> ("Value"=w1033:i32)  [unwired: 2 in, 2 out]
            n649 = property on="Z Step PV" class="DigNum (strict)"() -> ("Value"=w1032:i32)  [unwired: 2 in, 2 out]
            n650 = property on="Z Backlash" class="DigNum (strict)"() -> ("Value"=w1021:i32)  [unwired: 2 in, 2 out]
            n651 = Subtract(x=w1033, y=w1032) -> (x-y=w1031:i32)
            n652 = Sign(1:w1021) -> (0:w1029:i32)
            n653 = Sign(1:w1031) -> (0:w1030:i32)
            n654 = Multiply(x=w1030, y=w1029) -> (x*y=w1028:i32)
            n655 = Equal?(x=w1028, y=1) -> (x = y?=w1026:bool)
            n656 = case shown="True" w1026 {
              tunnel: w1025 -> [w1036 w1038]
              tunnel: w1024 -> [w1035 w1037]
              tunnel: [w1035 w1037] -> w1023
              tunnel: [w1036 w1038] -> w1022
              frame False {
                n657 = property on="Z Backlash corr" class="Bool (strict)"("Val(Sgnl)"=FALSE ("Value (Signaling)")) -> ()  [unwired: 2 in, 2 out]
              }
              frame True {
                n658 = property on="Z Backlash corr" class="Bool (strict)"("Val(Sgnl)"=TRUE ("Value (Signaling)")) -> ()  [unwired: 2 in, 2 out]
              }
            }
          }
          frame #2 {
            w1040 = 0.1 ("Delay Time (s)")
            n659 = property on="Z Velocity SP step/sec" class="DigNum (strict)"() -> ("Value"=w1047:i32)  [unwired: 2 in, 2 out]
            n660 = property on="Z steps/rev" class="DigNum (strict)"() -> ("Value"=w1046:u32)  [unwired: 2 in, 2 out]
            n661 = Divide(x=w1047, y=w1046) -> (x/y=w1048:dbl)
            n662 = Number To Fractional String(number=w1048) -> (F-format string=w1049:string)  [unwired: 3 in]
            n663 = call "Applied Send Command.vi"("error in (no error)"=w1044, "Extra"=w1049, "Command"=T1."Velocity Setting", "VISA resource name"=w1045) -> ("error out"=w1042:errorcluster, "VISA resource name out"=w1043:refnum<visa-resource-name>)  [unwired: 3 in, 1 out]
            n664 = call "Time Delay52"("error in (no error)"=w1042, "Delay Time (s)"=w1040) -> ("error out"=w1041:errorcluster)  [unwired: 9 in]
          }
          frame #3 {
            # "Move to Abs Position"
            n665 = property on="Z Step SP" class="DigNum (strict)"() -> ("Value"=w1059:i32)  [unwired: 2 in, 2 out]
            n666 = Number To Decimal String(number=w1059) -> (decimal integer string=w1056:string)  [unwired: 1 in]
            n667 = call "Applied Send Command.vi"("error in (no error)"=w1057, "Extra"=w1056, "Command"=T1."Distance or Position", "VISA resource name"=w1055) -> ("error out"=w1052:errorcluster, "VISA resource name out"=w1054:refnum<visa-resource-name>)  [unwired: 3 in, 1 out]
            n668 = call "Time Delay51"("error in (no error)"=w1052, "Delay Time (s)"=w1051) -> ("error out"=w1053:errorcluster)  [unwired: 9 in]
          }
          frame #4 {
            n669 = call "Applied Send Command.vi"("error in (no error)"=w1060, "Command"=T1."Feed to Position", "VISA resource name"=w1063) -> ("error out"=w1061:errorcluster, "VISA resource name out"=w1062:refnum<visa-resource-name>)  [unwired: 4 in, 1 out]
            n670 = call "Time Delay28"("error in (no error)"=w1061, "Delay Time (s)"=w1065) -> ("error out"=w1066:errorcluster)  [unwired: 9 in]
          }
        }
      }
      event "X Go": Mouse Up {
        n671 = event-data() -> ()  [unwired: 1 in, 7 out]
        n672 = flat-sequence {
          tunnel: [w1082] -> w1078
          tunnel: [w1081] -> w1077
          tunnel: w1076 -> [w1082]
          tunnel: w1075 -> [w1081]
          tunnel: [w1087] -> w1080
          tunnel: [w1086] -> w1079
          tunnel: w1078 -> [w1089]
          tunnel: w1077 -> [w1088]
          tunnel: [w1108] -> w1072
          tunnel: [w1105] -> w1070
          tunnel: w1080 -> [w1109]
          tunnel: w1079 -> [w1110]
          tunnel: [w1104] -> w1068
          tunnel: w1072 -> [w1117]
          tunnel: [w1116] -> w1071
          tunnel: w1070 -> [w1118]
          tunnel: [w1119] -> w1069
          tunnel: w1068 -> [w1115]
          tunnel: [w1115] -> w1067
          tunnel: w1071 -> [w1129]
          tunnel: w1069 -> [w1128]
          tunnel: [w1127] -> w1074
          tunnel: [w1126] -> w1073
          tunnel: w1067 -> [w1124]
          frame #0 {
            n673 = property on="Scan Go" class="Bool"("DisabledEnum"=T2."Disabled and Grayed Out" ("Disabled")) -> ()  [unwired: 2 in, 2 out]
            n674 = property on="X Go" class="Bool"("DisabledEnum"=T2."Disabled and Grayed Out" ("Disabled")) -> ()  [unwired: 2 in, 2 out]
          }
          frame #1 {
            n675 = property on="X Step SP" class="DigNum (strict)"() -> ("Value"=w1097:i32)  [unwired: 2 in, 2 out]
            n676 = property on="X Step PV" class="DigNum (strict)"() -> ("Value"=w1096:i32)  [unwired: 2 in, 2 out]
            n677 = property on="X Backlash" class="DigNum (strict)"() -> ("Value"=w1085:i32)  [unwired: 2 in, 2 out]
            n678 = Subtract(x=w1097, y=w1096) -> (x-y=w1095:i32)
            n679 = Sign(1:w1085) -> (0:w1093:i32)
            n680 = Sign(1:w1095) -> (0:w1094:i32)
            n681 = Multiply(x=w1094, y=w1093) -> (x*y=w1092:i32)
            n682 = Equal?(x=w1092, y=1) -> (x = y?=w1090:bool)
            n683 = case shown="True" w1090 {
              tunnel: w1089 -> [w1100 w1102]
              tunnel: w1088 -> [w1099 w1101]
              tunnel: [w1099 w1101] -> w1087
              tunnel: [w1100 w1102] -> w1086
              frame False {
                n684 = property on="X Backlash corr" class="Bool (strict)"("Val(Sgnl)"=FALSE ("Value (Signaling)")) -> ()  [unwired: 2 in, 2 out]
              }
              frame True {
                n685 = property on="X Backlash corr" class="Bool (strict)"("Val(Sgnl)"=TRUE ("Value (Signaling)")) -> ()  [unwired: 2 in, 2 out]
              }
            }
          }
          frame #2 {
            w1104 = 0.1 ("Delay Time (s)")
            n686 = property on="X Velocity SP step/sec" class="DigNum (strict)"() -> ("Value"=w1107:i32)  [unwired: 2 in, 2 out]
            n687 = property on="X steps/rev" class="DigNum (strict)"() -> ("Value"=w1111:u32)  [unwired: 2 in, 2 out]
            n688 = Divide(x=w1107, y=w1111) -> (x/y=w1112:dbl)
            n689 = Number To Fractional String(number=w1112) -> (F-format string=w1113:string)  [unwired: 3 in]
            n690 = call "Applied Send Command.vi"("error in (no error)"=w1109, "Extra"=w1113, "Command"=T1."Velocity Setting", "VISA resource name"=w1110) -> ("error out"=w1106:errorcluster, "VISA resource name out"=w1108:refnum<visa-resource-name>)  [unwired: 3 in, 1 out]
            n691 = call "Time Delay14"("error in (no error)"=w1106, "Delay Time (s)"=w1104) -> ("error out"=w1105:errorcluster)  [unwired: 9 in]
          }
          frame #3 {
            # "Distance/Position"
            n692 = property on="X Step SP" class="DigNum (strict)"() -> ("Value"=w1120:i32)  [unwired: 2 in, 2 out]
            n693 = Number To Decimal String(number=w1120) -> (decimal integer string=w1122:string)  [unwired: 1 in]
            n694 = call "Applied Send Command.vi"("error in (no error)"=w1118, "Extra"=w1122, "Command"=T1."Distance or Position", "VISA resource name"=w1117) -> ("error out"=w1121:errorcluster, "VISA resource name out"=w1116:refnum<visa-resource-name>)  [unwired: 3 in, 1 out]
            n695 = call "Time Delay31"("error in (no error)"=w1121, "Delay Time (s)"=w1115) -> ("error out"=w1119:errorcluster)  [unwired: 9 in]
          }
          frame #4 {
            # "Feed to Position"
            n696 = call "Applied Send Command.vi"("error in (no error)"=w1128, "Command"=T1."Feed to Position", "VISA resource name"=w1129) -> ("error out"=w1125:errorcluster, "VISA resource name out"=w1127:refnum<visa-resource-name>)  [unwired: 4 in, 1 out]
            n697 = call "Time Delay15"("error in (no error)"=w1125, "Delay Time (s)"=w1124) -> ("error out"=w1126:errorcluster)  [unwired: 9 in]
          }
        }
      }
      event "X Scan OK": Mouse Up {
        n698 = event-data() -> ()  [unwired: 1 in, 7 out]
        n699 = flat-sequence {
          tunnel: [w1146] -> w1138
          tunnel: [w1157] -> w1137
          tunnel: w1136 -> [w1154]
          tunnel: w1135 -> [w1153]
          tunnel: w1138 -> [w1164]
          tunnel: w1137 -> [w1163]
          tunnel: [w1164] -> w1132
          tunnel: [w1163] -> w1131
          tunnel: [w1166] -> w1133
          tunnel: [w1167] -> w1134
          tunnel: w1132 -> [w1167]
          tunnel: w1131 -> [w1166]
          frame #0 {
            # "VELOCITY"
            n700 = property on="X steps/rev" class="DigNum (strict)"() -> ("Value"=w1139:u32)  [unwired: 2 in, 2 out]
            n701 = property on="X Scan Velocity SP steps/sec" class="DigNum (strict)"() -> ("Value"=w1140:i32)  [unwired: 2 in, 2 out]
            n702 = Divide(x=w1140, y=w1139) -> (x/y=w1141:dbl)
            n703 = Number To Fractional String(number=w1141) -> (F-format string=w1155:string)  [unwired: 3 in]
            n704 = call "Applied Send Command.vi"("error in (no error)"=w1153, "Extra"=w1155, "Command"=T1."Velocity Setting", "VISA resource name"=w1154) -> ("error out"=w1142:errorcluster, "VISA resource name out"=w1143:refnum<visa-resource-name>)  [unwired: 3 in, 1 out]
            n705 = call "Time Delay9"("error in (no error)"=w1142) -> ("error out"=w1144:errorcluster)  [unwired: 10 in]
            n706 = call "Applied Send Command.vi"("error in (no error)"=w1144, "Extra"="", "Command"=T1."Velocity Setting", "VISA resource name"=w1143) -> ("error out"=w1145:errorcluster, "read buffer"=w1150:string, "VISA resource name out"=w1146:refnum<visa-resource-name>)  [unwired: 3 in]
            n707 = call "Time Delay10"("error in (no error)"=w1145) -> ("error out"=w1157:errorcluster)  [unwired: 10 in]
            n708 = Fract/Exp String To Number(string=w1150, offset=3) -> (number=w1148:dbl)  [unwired: 2 in, 1 out]
            n709 = Multiply(x=w1148, y=w1139) -> (x*y=w1147:dbl)
            n710 = property on="X velocity PV step/sec" class="DigNum (strict)"("Val(Sgnl)"=w1147) -> ()  [unwired: 2 in, 2 out]
          }
          frame #1 {
            n711 = property on="X Scan" class="Bool (strict)"("Val(Sgnl)"=TRUE ("Slew Ready 2")) -> ()  [unwired: 2 in, 2 out]
            n712 = property on="Scan Cancel" class="Bool"("DisabledEnum"=T2."Enabled" ("Disabled")) -> ()  [unwired: 2 in, 2 out]
            n713 = property on="Scan Go" class="Bool"("DisabledEnum"=T2."Enabled" ("Disabled")) -> ()  [unwired: 2 in, 2 out]
            n714 = property on="X Scan Length SP steps" class="DigNum (strict)"("DisabledEnum"=T2."Disabled and Grayed Out" ("Disabled")) -> ()  [unwired: 2 in, 2 out]
            n715 = property on="X Scan Velocity SP steps/sec" class="DigNum (strict)"("DisabledEnum"=T2."Disabled and Grayed Out" ("Disabled")) -> ()  [unwired: 2 in, 2 out]
          }
          frame #2 {
            n716 = property on="X Go" class="Bool"("DisabledEnum"=T2."Disabled and Grayed Out" ("Disabled")) -> ()  [unwired: 2 in, 2 out]
          }
        }
      }
      event "Y Scan OK": Mouse Up {
        n717 = event-data() -> ()  [unwired: 1 in, 7 out]
        n718 = flat-sequence {
          tunnel: w1175 -> [w1187]
          tunnel: w1174 -> [w1188]
          tunnel: [w1178] -> w1172
          tunnel: [w1194] -> w1171
          tunnel: w1172 -> [w1201]
          tunnel: w1171 -> [w1200]
          tunnel: [w1201] -> w1169
          tunnel: [w1200] -> w1168
          tunnel: [w1203] -> w1173
          tunnel: [w1204] -> w1170
          tunnel: w1169 -> [w1204]
          tunnel: w1168 -> [w1203]
          frame #0 {
            # "VELOCITY"
            n719 = property on="Y Scan Velocity SP steps/sec" class="DigNum (strict)"() -> ("Value"=w1190:i32)  [unwired: 2 in, 2 out]
            n720 = property on="Y steps/rev" class="DigNum (strict)"() -> ("Value"=w1181:u32)  [unwired: 2 in, 2 out]
            n721 = Divide(x=w1190, y=w1181) -> (x/y=w1191:dbl)
            n722 = Number To Fractional String(number=w1191) -> (F-format string=w1192:string)  [unwired: 3 in]
            n723 = call "Applied Send Command.vi"("error in (no error)"=w1187, "Extra"=w1192, "Command"=T1."Velocity Setting", "VISA resource name"=w1188) -> ("error out"=w1189:errorcluster, "VISA resource name out"=w1179:refnum<visa-resource-name>)  [unwired: 3 in, 1 out]
            n724 = call "Time Delay5"("error in (no error)"=w1189) -> ("error out"=w1180:errorcluster)  [unwired: 10 in]
            n725 = call "Applied Send Command.vi"("error in (no error)"=w1180, "Extra"="", "Command"=T1."Velocity Setting", "VISA resource name"=w1179) -> ("error out"=w1177:errorcluster, "read buffer"=w1184:string, "VISA resource name out"=w1178:refnum<visa-resource-name>)  [unwired: 3 in]
            n726 = Fract/Exp String To Number(string=w1184, offset=3) -> (number=w1183:dbl)  [unwired: 2 in, 1 out]
            n727 = call "Time Delay6"("error in (no error)"=w1177) -> ("error out"=w1194:errorcluster)  [unwired: 10 in]
            n728 = Multiply(x=w1183, y=w1181) -> (x*y=w1182:dbl)
            n729 = property on="Y velocity PV step/sec" class="DigNum (strict)"("Val(Sgnl)"=w1182) -> ()  [unwired: 2 in, 2 out]
          }
          frame #1 {
            n730 = property on="Y Scan" class="Bool (strict)"("Val(Sgnl)"=TRUE ("Slew Ready 2")) -> ()  [unwired: 2 in, 2 out]
            n731 = property on="Scan Cancel" class="Bool"("DisabledEnum"=T2."Enabled" ("Disabled")) -> ()  [unwired: 2 in, 2 out]
            n732 = property on="Scan Go" class="Bool"("DisabledEnum"=T2."Enabled" ("Disabled")) -> ()  [unwired: 2 in, 2 out]
            n733 = property on="Y Scan Length SP steps" class="DigNum (strict)"("DisabledEnum"=T2."Disabled and Grayed Out" ("Disabled")) -> ()  [unwired: 2 in, 2 out]
            n734 = property on="Y Scan Velocity SP steps/sec" class="DigNum (strict)"("DisabledEnum"=T2."Disabled and Grayed Out" ("Disabled")) -> ()  [unwired: 2 in, 2 out]
          }
          frame #2 {
            n735 = property on="Y Go" class="Bool"("DisabledEnum"=T2."Disabled and Grayed Out" ("Disabled")) -> ()  [unwired: 2 in, 2 out]
          }
        }
      }
      event "Z Scan OK": Mouse Up {
        n736 = event-data() -> ()  [unwired: 1 in, 7 out]
        n737 = flat-sequence {
          tunnel: [w1217] -> w1212
          tunnel: [w1231] -> w1211
          tunnel: w1208 -> [w1213]
          tunnel: w1207 -> [w1214]
          tunnel: w1212 -> [w1238]
          tunnel: w1211 -> [w1237]
          tunnel: [w1238] -> w1210
          tunnel: [w1237] -> w1209
          tunnel: [w1240] -> w1206
          tunnel: [w1241] -> w1205
          tunnel: w1210 -> [w1241]
          tunnel: w1209 -> [w1240]
          frame #0 {
            # "VELOCITY"
            n738 = property on="Z Scan Velocity SP steps/sec" class="DigNum (strict)"() -> ("Value"=w1227:i32)  [unwired: 2 in, 2 out]
            n739 = property on="Z steps/rev" class="DigNum (strict)"() -> ("Value"=w1220:u32)  [unwired: 2 in, 2 out]
            n740 = Divide(x=w1227, y=w1220) -> (x/y=w1228:dbl)
            n741 = Number To Fractional String(number=w1228) -> (F-format string=w1229:string)  [unwired: 3 in]
            n742 = call "Applied Send Command.vi"("error in (no error)"=w1214, "Extra"=w1229, "Command"=T1."Velocity Setting", "VISA resource name"=w1213) -> ("error out"=w1226:errorcluster, "VISA resource name out"=w1216:refnum<visa-resource-name>)  [unwired: 3 in, 1 out]
            n743 = call "Time Delay24"("error in (no error)"=w1226) -> ("error out"=w1215:errorcluster)  [unwired: 10 in]
            n744 = call "Applied Send Command.vi"("error in (no error)"=w1215, "Extra"="", "Command"=T1."Velocity Setting", "VISA resource name"=w1216) -> ("error out"=w1218:errorcluster, "read buffer"=w1223:string, "VISA resource name out"=w1217:refnum<visa-resource-name>)  [unwired: 3 in]
            n745 = call "Time Delay25"("error in (no error)"=w1218) -> ("error out"=w1231:errorcluster)  [unwired: 10 in]
            n746 = Fract/Exp String To Number(string=w1223, offset=3) -> (number=w1222:dbl)  [unwired: 2 in, 1 out]
            n747 = Multiply(x=w1222, y=w1220) -> (x*y=w1219:dbl)
            n748 = property on="Z  velocity PV step/sec" class="DigNum (strict)"("Val(Sgnl)"=w1219) -> ()  [unwired: 2 in, 2 out]
          }
          frame #1 {
            n749 = property on="Z Scan" class="Bool (strict)"("Val(Sgnl)"=TRUE ("Slew Ready 2")) -> ()  [unwired: 2 in, 2 out]
            n750 = property on="Scan Cancel" class="Bool"("DisabledEnum"=T2."Enabled" ("Disabled")) -> ()  [unwired: 2 in, 2 out]
            n751 = property on="Scan Go" class="Bool"("DisabledEnum"=T2."Enabled" ("Disabled")) -> ()  [unwired: 2 in, 2 out]
            n752 = property on="Z Scan Length SP steps" class="DigNum (strict)"("DisabledEnum"=T2."Disabled and Grayed Out" ("Disabled")) -> ()  [unwired: 2 in, 2 out]
            n753 = property on="Z Scan Velocity SP steps/sec" class="DigNum (strict)"("DisabledEnum"=T2."Disabled and Grayed Out" ("Disabled")) -> ()  [unwired: 2 in, 2 out]
          }
          frame #2 {
            n754 = property on="Z Go" class="Bool"("DisabledEnum"=T2."Disabled and Grayed Out" ("Disabled")) -> ()  [unwired: 2 in, 2 out]
          }
        }
      }
      event Application Instance Close? {
        n755 = event-data() -> ()  [unwired: 1 in, 4 out]
        n756 = event-data() -> ()  [unwired: 3 in, 1 out]
      }
      event "Stop": Mouse Down {
        n757 = event-data() -> ()  [unwired: 1 in, 7 out]
        n758 = flat-sequence {
          tunnel: [w1263] -> w1251
          tunnel: [w1262] -> w1250
          tunnel: w1249 -> [w1264]
          tunnel: w1248 -> [w1261]
          frame #0 {
            n759 = call "Applied Send Command.vi"("error in (no error)"=w1261, "Command"=T1."Stop", "VISA resource name"=w1264) -> ("error out"=w1262:errorcluster, "VISA resource name out"=w1263:refnum<visa-resource-name>)  [unwired: 4 in, 1 out]
          }
        }
        n760 = flat-sequence {
          tunnel: w1255 -> [w1267]
          tunnel: w1254 -> [w1266]
          tunnel: [w1268] -> w1253
          tunnel: [w1269] -> w1252
          frame #0 {
            n761 = call "Applied Send Command.vi"("error in (no error)"=w1266, "Command"=T1."Stop", "VISA resource name"=w1267) -> ("error out"=w1269:errorcluster, "VISA resource name out"=w1268:refnum<visa-resource-name>)  [unwired: 4 in, 1 out]
          }
        }
        n762 = flat-sequence {
          tunnel: [w1258] -> w1245
          tunnel: [w1259] -> w1244
          tunnel: w1247 -> [w1256]
          tunnel: w1246 -> [w1257]
          frame #0 {
            n763 = call "Applied Send Command.vi"("error in (no error)"=w1257, "Command"=T1."Stop", "VISA resource name"=w1256) -> ("error out"=w1259:errorcluster, "VISA resource name out"=w1258:refnum<visa-resource-name>)  [unwired: 4 in, 1 out]
          }
        }
      }
      event "Scan Cancel": Mouse Down {
        n764 = event-data() -> ()  [unwired: 1 in, 7 out]
        n765 = flat-sequence {
          tunnel: w1280 -> [w1305]
          tunnel: w1279 -> [w1304]
          tunnel: [w1307] -> w1282
          tunnel: [w1306] -> w1281
          tunnel: [w1315] -> w1277
          tunnel: [w1316] -> w1278
          tunnel: w1282 -> [w1316]
          tunnel: w1281 -> [w1315]
          frame #0 {
            n766 = call "Applied Send Command.vi"("error in (no error)"=w1304, "Command"=T1."Stop", "VISA resource name"=w1305) -> ("error out"=w1306:errorcluster, "VISA resource name out"=w1307:refnum<visa-resource-name>)  [unwired: 4 in, 1 out]
          }
          frame #1 {
            n767 = property on="X Scan" class="Bool (strict)"("Value"=FALSE ("Slew Ready")) -> ()  [unwired: 2 in, 2 out]
            n768 = property on="X Scan set" class="Bool"("DisabledEnum"=T2."Enabled" ("Disabled")) -> ()  [unwired: 2 in, 2 out]
            n769 = property on="X Scan Velocity SP steps/sec" class="DigNum (strict)"("DisabledEnum"=T2."Enabled" ("Disabled")) -> ()  [unwired: 2 in, 2 out]
            n770 = property on="X Scan Length SP steps" class="DigNum (strict)"("DisabledEnum"=T2."Enabled" ("Disabled")) -> ()  [unwired: 2 in, 2 out]
            n771 = property on="X Go" class="Bool"("DisabledEnum"=T2."Enabled" ("Disabled")) -> ()  [unwired: 2 in, 2 out]
            n772 = property on="X Scan OK" class="Bool"("DisabledEnum"=T2."Enabled" ("Disabled")) -> ()  [unwired: 2 in, 2 out]
          }
        }
        n773 = flat-sequence {
          tunnel: w1288 -> [w1318]
          tunnel: w1287 -> [w1317]
          tunnel: [w1320] -> w1284
          tunnel: [w1319] -> w1283
          tunnel: [w1328] -> w1289
          tunnel: [w1329] -> w1290
          tunnel: w1284 -> [w1329]
          tunnel: w1283 -> [w1328]
          frame #0 {
            n774 = call "Applied Send Command.vi"("error in (no error)"=w1317, "Command"=T1."Stop", "VISA resource name"=w1318) -> ("error out"=w1319:errorcluster, "VISA resource name out"=w1320:refnum<visa-resource-name>)  [unwired: 4 in, 1 out]
          }
          frame #1 {
            n775 = property on="Y Scan" class="Bool (strict)"("Value"=FALSE ("Slew Ready")) -> ()  [unwired: 2 in, 2 out]
            n776 = property on="Y Go" class="Bool"("DisabledEnum"=T2."Enabled" ("Disabled")) -> ()  [unwired: 2 in, 2 out]
            n777 = property on="Y Scan Velocity SP steps/sec" class="DigNum (strict)"("DisabledEnum"=T2."Enabled" ("Disabled")) -> ()  [unwired: 2 in, 2 out]
            n778 = property on="Y Scan set" class="Bool"("DisabledEnum"=T2."Enabled" ("Disabled")) -> ()  [unwired: 2 in, 2 out]
            n779 = property on="Y Scan OK" class="Bool"("DisabledEnum"=T2."Enabled" ("Disabled")) -> ()  [unwired: 2 in, 2 out]
            n780 = property on="Y Scan Length SP steps" class="DigNum (strict)"("DisabledEnum"=T2."Enabled" ("Disabled")) -> ()  [unwired: 2 in, 2 out]
          }
        }
        n781 = flat-sequence {
          tunnel: [w1294] -> w1276
          tunnel: [w1293] -> w1275
          tunnel: w1274 -> [w1292]
          tunnel: w1273 -> [w1291]
          tunnel: [w1302] -> w1271
          tunnel: [w1303] -> w1272
          tunnel: w1276 -> [w1303]
          tunnel: w1275 -> [w1302]
          frame #0 {
            n782 = call "Applied Send Command.vi"("error in (no error)"=w1291, "Command"=T1."Stop", "VISA resource name"=w1292) -> ("error out"=w1293:errorcluster, "VISA resource name out"=w1294:refnum<visa-resource-name>)  [unwired: 4 in, 1 out]
          }
          frame #1 {
            n783 = property on="Z Scan" class="Bool (strict)"("Value"=FALSE ("Slew Ready")) -> ()  [unwired: 2 in, 2 out]
            n784 = property on="Z Scan set" class="Bool"("DisabledEnum"=T2."Enabled" ("Disabled")) -> ()  [unwired: 2 in, 2 out]
            n785 = property on="Z Scan Velocity SP steps/sec" class="DigNum (strict)"("DisabledEnum"=T2."Enabled" ("Disabled")) -> ()  [unwired: 2 in, 2 out]
            n786 = property on="Z Scan Length SP steps" class="DigNum (strict)"("DisabledEnum"=T2."Enabled" ("Disabled")) -> ()  [unwired: 2 in, 2 out]
            n787 = property on="Z Go" class="Bool"("DisabledEnum"=T2."Enabled" ("Disabled")) -> ()  [unwired: 2 in, 2 out]
            n788 = property on="Z Scan OK" class="Bool"("DisabledEnum"=T2."Enabled" ("Disabled")) -> ()  [unwired: 2 in, 2 out]
          }
        }
        n789 = property on="Scan Go" class="Bool"("DisabledEnum"=T2."Disabled and Grayed Out" ("Disabled")) -> ()  [unwired: 2 in, 2 out]
        n790 = property on="Scan Cancel" class="Bool"("DisabledEnum"=T2."Disabled and Grayed Out" ("Disabled")) -> ()  [unwired: 2 in, 2 out]
      }
      event "Scan Go": Mouse Up {
        n791 = event-data() -> ()  [unwired: 1 in, 7 out]
        n792 = flat-sequence {
          tunnel: w1356 -> [w1370]
          tunnel: w1355 -> [w1371]
          tunnel: w1354 -> [w1368]
          tunnel: w1353 -> [w1369]
          tunnel: w1352 -> [w1367]
          tunnel: w1351 -> [w1366]
          tunnel: [w1365] -> w1344
          tunnel: [w1364] -> w1342
          tunnel: [w1363] -> w1340
          tunnel: [w1362] -> w1338
          tunnel: [w1361] -> w1336
          tunnel: [w1360] -> w1334
          tunnel: [w1359] -> w1332
          tunnel: [w1358] -> w1331
          tunnel: [w1357] -> w1330
          tunnel: w1344 -> [w1413]
          tunnel: [w1412] -> w1343
          tunnel: w1342 -> [w1411]
          tunnel: [w1410] -> w1341
          tunnel: w1340 -> [w1409]
          tunnel: [w1408] -> w1339
          tunnel: w1338 -> [w1407]
          tunnel: [w1406] -> w1337
          tunnel: w1336 -> [w1405]
          tunnel: [w1404] -> w1335
          tunnel: w1334 -> [w1402]
          tunnel: [w1403] -> w1333
          tunnel: w1332 -> [w1401]
          tunnel: w1331 -> [w1400]
          tunnel: w1330 -> [w1399]
          tunnel: [w1439] -> w1350
          tunnel: [w1438] -> w1349
          tunnel: [w1437] -> w1348
          tunnel: [w1436] -> w1347
          tunnel: [w1441] -> w1346
          tunnel: [w1440] -> w1345
          tunnel: w1343 -> [w1441]
          tunnel: w1341 -> [w1440]
          tunnel: w1339 -> [w1439]
          tunnel: w1337 -> [w1438]
          tunnel: w1335 -> [w1437]
          tunnel: w1333 -> [w1436]
          frame #0 {
            n793 = property on="X Scan" class="Bool (strict)"() -> ("Value"=w1357:bool)  [unwired: 2 in, 2 out]
            n794 = property on="Y Scan" class="Bool (strict)"() -> ("Value"=w1358:bool)  [unwired: 2 in, 2 out]
            n795 = property on="Z Scan" class="Bool (strict)"() -> ("Value"=w1359:bool)  [unwired: 2 in, 2 out]
            n796 = case shown="True" w1357 {
              tunnel: w1371 -> [w1382 w1386]
              tunnel: [w1382 w1385] -> w1364
              tunnel: w1370 -> [w1381 w1384]
              tunnel: [w1381 w1383] -> w1365
              frame False {
              }
              frame True {
                n797 = property on="X Scan Length SP steps" class="DigNum (strict)"() -> ("Value"=w1387:i32)  [unwired: 2 in, 2 out]
                n798 = Number To Decimal String(number=w1387) -> (decimal integer string=w1388:string)  [unwired: 1 in]
                n799 = call "Applied Send Command.vi"("error in (no error)"=w1386, "Extra"=w1388, "Command"=T1."Distance or Position", "VISA resource name"=w1384) -> ("error out"=w1385:errorcluster, "VISA resource name out"=w1383:refnum<visa-resource-name>)  [unwired: 3 in, 1 out]
              }
            }
            n800 = case shown="True" w1358 {
              tunnel: w1368 -> [w1391 w1396]
              tunnel: w1369 -> [w1390 w1395]
              tunnel: [w1390 w1392] -> w1362
              tunnel: [w1391 w1393] -> w1363
              frame False {
              }
              frame True {
                n801 = property on="Y Scan Length SP steps" class="DigNum (strict)"() -> ("Value"=w1394:i32)  [unwired: 2 in, 2 out]
                n802 = Number To Decimal String(number=w1394) -> (decimal integer string=w1397:string)  [unwired: 1 in]
                n803 = call "Applied Send Command.vi"("error in (no error)"=w1395, "Extra"=w1397, "Command"=T1."Distance or Position", "VISA resource name"=w1396) -> ("error out"=w1392:errorcluster, "VISA resource name out"=w1393:refnum<visa-resource-name>)  [unwired: 3 in, 1 out]
              }
            }
            n804 = case shown="True" w1359 {
              tunnel: w1367 -> [w1373 w1377]
              tunnel: [w1373 w1376] -> w1361
              tunnel: [w1372 w1375] -> w1360
              tunnel: w1366 -> [w1372 w1374]
              frame False {
              }
              frame True {
                n805 = property on="Z Scan Length SP steps" class="DigNum (strict)"() -> ("Value"=w1378:i32)  [unwired: 2 in, 2 out]
                n806 = Number To Decimal String(number=w1378) -> (decimal integer string=w1379:string)  [unwired: 1 in]
                n807 = call "Applied Send Command.vi"("error in (no error)"=w1374, "Extra"=w1379, "Command"=T1."Distance or Position", "VISA resource name"=w1377) -> ("error out"=w1375:errorcluster, "VISA resource name out"=w1376:refnum<visa-resource-name>)  [unwired: 3 in, 1 out]
              }
            }
          }
          frame #1 {
            n808 = case shown="True" w1399 {
              tunnel: w1413 -> [w1429 w1433]
              tunnel: [w1429 w1432] -> w1412
              tunnel: w1411 -> [w1428 w1431]
              tunnel: [w1428 w1430] -> w1410
              frame False {
              }
              frame True {
                n809 = call "Applied Send Command.vi"("error in (no error)"=w1431, "Command"=T1."Feed to Length", "VISA resource name"=w1433) -> ("error out"=w1430:errorcluster, "VISA resource name out"=w1432:refnum<visa-resource-name>)  [unwired: 4 in, 1 out]
              }
            }
            n810 = case shown="True" w1400 {
              tunnel: w1409 -> [w1422 w1426]
              tunnel: [w1422 w1425] -> w1408
              tunnel: w1407 -> [w1421 w1424]
              tunnel: [w1421 w1423] -> w1406
              frame False {
              }
              frame True {
                n811 = call "Applied Send Command.vi"("error in (no error)"=w1424, "Command"=T1."Feed to Length", "VISA resource name"=w1426) -> ("error out"=w1423:errorcluster, "VISA resource name out"=w1425:refnum<visa-resource-name>)  [unwired: 4 in, 1 out]
              }
            }
            n812 = case shown="False" w1401 {
              tunnel: w1405 -> [w1415 w1419]
              tunnel: [w1415 w1418] -> w1404
              tunnel: [w1414 w1417] -> w1403
              tunnel: w1402 -> [w1414 w1416]
              frame False {
              }
              frame True {
                n813 = call "Applied Send Command.vi"("error in (no error)"=w1416, "Command"=T1."Feed to Length", "VISA resource name"=w1419) -> ("error out"=w1417:errorcluster, "VISA resource name out"=w1418:refnum<visa-resource-name>)  [unwired: 4 in, 1 out]
              }
            }
          }
          frame #2 {
            (unwired) FALSE ("Slew Ready 2")
            n814 = call "Time Delay7"("Delay Time (s)"=0.1) -> ()  [unwired: 10 in, 1 out]
            n815 = property on="Z Scan" class="Bool (strict)"("Val(Sgnl)"=FALSE ("Slew Ready 2")) -> ()  [unwired: 2 in, 2 out]
            n816 = property on="X Scan" class="Bool (strict)"("Val(Sgnl)"=FALSE ("Slew Ready 2")) -> ()  [unwired: 2 in, 2 out]
            n817 = property on="Y Scan" class="Bool (strict)"("Val(Sgnl)"=FALSE ("Slew Ready 2")) -> ()  [unwired: 2 in, 2 out]
            n818 = property on="Z Scan Velocity SP steps/sec" class="DigNum (strict)"("DisabledEnum"=T2."Enabled" ("Disabled")) -> ()  [unwired: 2 in, 2 out]
            n819 = property on="X Scan Length SP steps" class="DigNum (strict)"("DisabledEnum"=T2."Enabled" ("Disabled")) -> ()  [unwired: 2 in, 2 out]
            n820 = property on="Y Scan Selocity SP steps/sec" class="DigNum (strict)"("DisabledEnum"=T2."Enabled" ("Disabled")) -> ()  [unwired: 2 in, 2 out]
            n821 = property on="Z Scan Length SP steps" class="DigNum (strict)"("DisabledEnum"=T2."Enabled" ("Disabled")) -> ()  [unwired: 2 in, 2 out]
            n822 = property on="Y Scan Length SP steps" class="DigNum (strict)"("DisabledEnum"=T2."Enabled" ("Disabled")) -> ()  [unwired: 2 in, 2 out]
            n823 = property on="X Scan Velocity SP steps/sec" class="DigNum (strict)"("DisabledEnum"=T2."Enabled" ("Disabled")) -> ()  [unwired: 2 in, 2 out]
            n824 = property on="Scan Go" class="Bool"("DisabledEnum"=T2."Disabled and Grayed Out" ("Disabled")) -> ()  [unwired: 2 in, 2 out]
            n825 = property on="Scan Cancel" class="Bool"("DisabledEnum"=T2."Disabled and Grayed Out" ("Disabled")) -> ()  [unwired: 2 in, 2 out]
          }
        }
      }
      event "Reset": Mouse Down {
        n826 = event-data() -> ()  [unwired: 1 in, 7 out]
        n827 = flat-sequence {
          tunnel: [w1472] -> w1458
          tunnel: w1459 -> [w1474]
          tunnel: [w1473] -> w1457
          tunnel: w1460 -> [w1475]
          frame #0 {
            n828 = property on="Reset X Motor Steps" class="DigNum (strict)"() -> ("Value"=w1478:i32)  [unwired: 2 in, 2 out]
            n829 = Number To Decimal String(number=w1478) -> (decimal integer string=w1476:string)  [unwired: 1 in]
            n830 = call "Applied Send Command.vi"("error in (no error)"=w1474, "Extra"=w1476, "Command"=T1."Set ABS Position", "VISA resource name"=w1475) -> ("error out"=w1473:errorcluster, "VISA resource name out"=w1472:refnum<visa-resource-name>)  [unwired: 3 in, 1 out]
          }
        }
        n831 = flat-sequence {
          tunnel: w1464 -> [w1483]
          tunnel: w1463 -> [w1480]
          tunnel: [w1482] -> w1462
          tunnel: [w1481] -> w1461
          frame #0 {
            n832 = property on="Reset Y Motor Steps" class="DigNum (strict)"() -> ("Value"=w1485:i32)  [unwired: 2 in, 2 out]
            n833 = Number To Decimal String(number=w1485) -> (decimal integer string=w1484:string)  [unwired: 1 in]
            n834 = call "Applied Send Command.vi"("error in (no error)"=w1480, "Extra"=w1484, "Command"=T1."Set ABS Position", "VISA resource name"=w1483) -> ("error out"=w1481:errorcluster, "VISA resource name out"=w1482:refnum<visa-resource-name>)  [unwired: 3 in, 1 out]
          }
        }
        n835 = flat-sequence {
          tunnel: [w1470] -> w1454
          tunnel: [w1469] -> w1453
          tunnel: w1456 -> [w1467]
          tunnel: w1455 -> [w1468]
          frame #0 {
            n836 = property on="Reset Z Motor Steps" class="DigNum (strict)"() -> ("Value"=w1471:i32)  [unwired: 2 in, 2 out]
            n837 = Number To Decimal String(number=w1471) -> (decimal integer string=w1465:string)  [unwired: 1 in]
            n838 = call "Applied Send Command.vi"("error in (no error)"=w1468, "Extra"=w1465, "Command"=T1."Set ABS Position", "VISA resource name"=w1467) -> ("error out"=w1469:errorcluster, "VISA resource name out"=w1470:refnum<visa-resource-name>)  [unwired: 3 in, 1 out]
          }
        }
      }
    }
    n839 = case shown="True" "Delete Button" {
      tunnel: w287 -> [_ w310]
      frame False {
      }
      frame True {
        n840 = property on="Preset positions" class="Ring (strict)"() -> ("Value"=w308:i32)  [unwired: 2 in, 2 out]
        n841 = Delete From Array(array=w310, index=w308) -> (array with subset deleted=w309:string[])  [unwired: 1 in, 1 out]
        n842 = property on="Presets" class="Arr (strict)"() -> ("Value"=w307:i32[][])  [unwired: 2 in, 2 out]
        n843 = property on="Preset positions" class="Ring (strict)"("Strings []"=w309) -> ()  [unwired: 2 in, 2 out]
        n844 = Delete From Array(array=w307, index (row)=w308) -> (array with subset deleted=w306:i32[][])  [unwired: 2 in, 1 out]
        n845 = property on="Presets" class="Arr (strict)"("Val(Sgnl)"=w306) -> ()  [unwired: 2 in, 2 out]
      }
    }
    n846 = case shown="True" "Set Button" {
      tunnel: "Preset positions" -> [_ w326]
      frame False {
      }
      frame True {
        n847 = property on="Presets" class="Arr (strict)"() -> ("Value"=w323:i32[][])  [unwired: 2 in, 2 out]
        n848 = Index Array(array=w323, index (row)=w326) -> (element=w325:i32[])  [unwired: 1 in]
        n849 = Array To Cluster(array=w325) -> (cluster=w324:T4)
        n850 = Unbundle(w324) -> ("Value[0]"=w322:i32, "Value[1]"=w321:i32, "Value[2]"=w320:i32)  [unwired: 6 out]
        n851 = property on="X Step SP" class="DigNum (strict)"("Val(Sgnl)"=w322) -> ()  [unwired: 2 in, 2 out]
        n852 = property on="Y Step SP" class="DigNum (strict)"("Val(Sgnl)"=w321) -> ()  [unwired: 2 in, 2 out]
        n853 = property on="Z Step SP" class="DigNum (strict)"("Val(Sgnl)"=w320) -> ()  [unwired: 2 in, 2 out]
      }
    }
    n854 = case shown="True" "Add Button" {
      tunnel: w287 -> [_ w319]
      frame False {
      }
      frame True {
        n855 = property on="X Step PV" class="DigNum (strict)"() -> ("Value"=w314:i32)  [unwired: 2 in, 2 out]
        n856 = property on="Y Step PV" class="DigNum (strict)"() -> ("Value"=w313:i32)  [unwired: 2 in, 2 out]
        n857 = property on="Z Step PV" class="DigNum (strict)"() -> ("Value"=w312:i32)  [unwired: 2 in, 2 out]
        n858 = Build Array(w314, w313, w312) -> (w317:i32[])
        n859 = Build Array (concatenate)(w319, "String") -> (w318:string[])
        n860 = property on="Preset positions" class="Ring (strict)"("Strings []"=w318) -> ()  [unwired: 2 in, 2 out]
        n861 = property on="Presets" class="Arr (strict)"() -> ("Value"=w316:i32[][])  [unwired: 2 in, 2 out]
        n862 = Build Array (concatenate)(w316, w317) -> (w311:i32[][])
        n863 = property on="Presets" class="Arr (strict)"("Val(Sgnl)"=w311) -> ()  [unwired: 2 in, 2 out]
      }
    }
  }
  n864 = flat-sequence {
    tunnel: w55 -> [w1487]
    tunnel: w54 -> [w1486]
    tunnel: [w1498] -> w39
    frame #0 {
      # "GET CURRENT POSITION"
      n865 = call "Applied Send Command.vi"("error in (no error)"=w1486, "Extra"="", "Command"=T1."Immediate Position?", "VISA resource name"=w1487) -> ("error out"=w1488:errorcluster, "read buffer"=w1493:string, "VISA resource name out"=w1489:refnum<visa-resource-name>)  [unwired: 3 in]
      n866 = call "Applied Send Command.vi"("error in (no error)"=w1488, "Command"=T1."Stop & Kill Buffer", "VISA resource name"=w1489) -> ("error out"=w1495:errorcluster, "VISA resource name out"=w1496:refnum<visa-resource-name>)  [unwired: 4 in, 1 out]
      n867 = Hexadecimal String To Number(string=w1493, offset=3) -> (number=w1490:u32)  [unwired: 1 in, 1 out]
      n868 = VISA Close(VISA resource name=w1496, error in (no error)=w1495) -> ()  [unwired: 1 out]
      n869 = To Long Integer(number=w1490) -> (32bit integer=w1498:i32)
    }
  }
  n870 = flat-sequence {
    tunnel: w41 -> [w1501]
    tunnel: w40 -> [w1500]
    tunnel: [w1499] -> w38
    frame #0 {
      # "GET CURRENT POSITION"
      n871 = call "Applied Send Command.vi"("error in (no error)"=w1500, "Extra"="", "Command"=T1."Immediate Position?", "VISA resource name"=w1501) -> ("error out"=w1502:errorcluster, "read buffer"=w1507:string, "VISA resource name out"=w1503:refnum<visa-resource-name>)  [unwired: 3 in]
      n872 = call "Applied Send Command.vi"("error in (no error)"=w1502, "Command"=T1."Stop & Kill Buffer", "VISA resource name"=w1503) -> ("error out"=w1509:errorcluster, "VISA resource name out"=w1510:refnum<visa-resource-name>)  [unwired: 4 in, 1 out]
      n873 = Hexadecimal String To Number(string=w1507, offset=3) -> (number=w1504:u32)  [unwired: 1 in, 1 out]
      n874 = VISA Close(VISA resource name=w1510, error in (no error)=w1509) -> ()  [unwired: 1 out]
      n875 = To Long Integer(number=w1504) -> (32bit integer=w1499:i32)
    }
  }
  n876 = flat-sequence {
    tunnel: w43 -> [w1513]
    tunnel: w42 -> [w1512]
    tunnel: [w1514] -> w37
    frame #0 {
      # "GET CURRENT POSITION"
      n877 = call "Applied Send Command.vi"("error in (no error)"=w1512, "Extra"="", "Command"=T1."Immediate Position?", "VISA resource name"=w1513) -> ("error out"=w1515:errorcluster, "read buffer"=w1520:string, "VISA resource name out"=w1516:refnum<visa-resource-name>)  [unwired: 3 in]
      n878 = call "Applied Send Command.vi"("error in (no error)"=w1515, "Command"=T1."Stop & Kill Buffer", "VISA resource name"=w1516) -> ("error out"=w1522:errorcluster, "VISA resource name out"=w1523:refnum<visa-resource-name>)  [unwired: 4 in, 1 out]
      n879 = Hexadecimal String To Number(string=w1520, offset=3) -> (number=w1517:u32)  [unwired: 1 in, 1 out]
      n880 = VISA Close(VISA resource name=w1523, error in (no error)=w1522) -> ()  [unwired: 1 out]
      n881 = To Long Integer(number=w1517) -> (32bit integer=w1514:i32)
    }
  }
  n882 = flat-sequence {
    tunnel: w39 -> [w1529]
    tunnel: w38 -> [w1528]
    tunnel: w37 -> [w1527]
    frame #0 {
      n883 = Build Array(w1529, w1528, w1527) -> (w1525:i32[])
      n884 = call-poly <vilib>:"Write To Spreadsheet File.vi"("1D data"=w1525, "file path (dialog if empty)"=path "S:/SSE/SCL2/POS.TXT") -> ()  [unwired: 6 in, 1 out]
    }
    frame #1 {
      n885 = property on="Presets" class="Arr (strict)"() -> ("Value"=w1536:i32[][])  [unwired: 2 in, 2 out]
      n886 = property on="Preset positions" class="Ring (strict)"() -> ("Strings []"=w1532:string[])  [unwired: 2 in, 2 out]
      n887 = Number To Decimal String(number=w1536) -> (decimal integer string=w1530:string[][])  [unwired: 1 in]
      n888 = Transpose 2D Array(2D array=w1530) -> (transposed array=w1531:string[][])
      n889 = Build Array (concatenate)(w1532, w1531) -> (w1533:string[][])
      n890 = Transpose 2D Array(2D array=w1533) -> (transposed array=w1534:string[][])
      n891 = call-poly <vilib>:"Write To Spreadsheet File.vi"("2D data"=w1534, "file path (dialog if empty)"=path "S:/SSE/SCL2/PRESET.TXT") -> ()  [unwired: 6 in, 1 out]
    }
  }
